vi "Insert2012.vi"(6 "Variant in":variant, 7 "Shift Pressed?":bool, 8 "error in (no error)":errorcluster, 10 "QD Combo Box Ref":refnum<vi>, 11 "QD Launch VI Ref":refnum<vi>) -> (0 "error out":errorcluster, 4 "Variant out":variant)   [LabVIEW 2012]
doc: "Inserts the object specified by name in the Quick Drop dialog box on the selected wire(s) on the diagram. If [Shift] is also pressed, and multiple wires were selected, a single instance of the object is inserted on those wires.\n\nDefault Shortcut - [I]"
uses:
  <vilib>/Utility/miscctls.llb/LVPositionTypeDef.ctl
  <vilib>/Utility/miscctls.llb/LVPointTypeDef.ctl
panel:
  in  "Style":i32(ring)=2125 items=[".NET Container"=2125, ".NET Refnum"=3441, "2D Picture"=3508, "3D Picture"=23776, "Absolute Value"=1054, "Access Rights"=1412, "ActiveX Container"=2072, "Add"=1050, "Add (with error terminals)"=3915, "Add Array Elements"=1903, "Agitator"=3831, "AllSpoll"=1960, "Always Copy"=2400, "And"=1061, "And Array Elements"=1911, "Append True/False String"=1511, "Application Refnum"=3412, "Array (block diagram constant)"=2070, "Array (classic)"=3300, "Array (modern)"=21608, "Array Interface Control"=23777, "Array Max & Min"=1907, "Array of Strings to Path"=1422, "Array Size"=1809, "Array Subset"=2044, "Array To Cluster"=1168, "Array To Spreadsheet String"=1540, "Atmospheric Tank (classic)"=3070, "Atmospheric Tank (modern)"=21751, "Automation Close"=8001, "Automation Open"=8000, "Automation Refnum"=3410, "Avogadro Constant (1/mol)"=23520, "Base 10 Logarithm Of e"=23512, "Bin #1"=3073, "Bin #2"=21755, "Bitpack to Array"=3135, "Bluetooth Close Connection"=9148, "Bluetooth Create Listener"=9151, "Bluetooth Discover"=9152, "Bluetooth Network Connection Refnum"=3468, "Bluetooth Open Connection"=9153, "Bluetooth Read"=9149, "Bluetooth Wait On Listener"=9147, "Bluetooth Write"=9150, "Boolean Array To Number"=1815, "Boolean To (0,1)"=1167, "Build Array"=2041, "Build Cluster Array"=2047, "Build Matrix"=8500, "Build Path"=1419, "Build Waveform"=2066, "Bundle"=2049, "Bundle By Name"=2057, "Byte Array To String"=1609, "Byte Stream File Refnum"=3408, "Call By Reference"=3901, "Call Chain"=1999, "Call Library Function Node"=2062, "Call Parent Method"=2354, "CAN Channel (block diagram constant)"=2124, "CAN Channel (classic)"=3340, "CAN Channel (modern)"=21817, "CAN Channel (system)"=21966, "CAN Interface (block diagram constant)"=2123, "CAN Interface (classic)"=3339, "CAN Interface (modern)"=21815, "CAN Interface (system)"=21964, "CAN Task (block diagram constant)"=3471, "CAN Task (classic)"=3470, "CAN Task (modern)"=21789, "CAN Task (system)"=21963, "Cancel Button (modern)"=21739, "Cancel Button (system)"=3131, "Cancel Notification"=9107, "Carriage Return Constant"=23500, "Case Structure"=2001, "Cast Unit Bases"=1079, "Check Valve"=3833, "Checkbox (classic)"=3117, "CheckBox (modern)"=21924, "Checkbox (system)"=3132, "Class Specifier Constant"=2094, "Clear Fixed-Point Overflow Status"=5562, "Close File"=8052, "Close File (deprecated)"=1405, "Close Reference"=8011, "Close Variable Connection"=23783, "Cluster (classic)"=3400, "Cluster (modern)"=21607, "Cluster Constant"=2071, "Cluster To Array"=1169, "Code Interface Node"=2050, "Coerce To Type"=2402, "Color Box"=3013, "Color Box Constant"=2120, "Color Box Thin Border"=2905, "Color Ramp"=3022, "Colored Rectangle (broken?)"=3625, "Combo Box (classic)"=3304, "Combo Box (modern)"=21604, "Combo Box (system)"=21917, "Combo Box Constant"=2088, "Complex Conjugate"=1048, "Complex To Polar"=1045, "Complex To Re/Im"=1044, "Compound Arithmetic"=2200, "Compressor"=3832, "Concatenate Strings"=2040, "Conditional Disable Structure"=2064, "Constructor Node"=3904, "Control & Simulation Loop"=2099, "Control Help Window"=1353, "Control Online Help"=1355, "Control Refnum"=3419, "Convert Unit"=2059, "Conveyer"=3827, "Copy"=8053, "Copy (deprecated)"=1416, "Cosecant"=1204, "Cosine"=1201, "Cotangent"=1205, "CPU Information"=24130, "Create Folder"=8055, "Create Network Stream Endpoint"=23793, "Create Network Stream Reader Endpoint"=23811, "Create Network Stream Writer Endpoint"=23810, "Create Stream"=23796, "Create Unique Network Stream Endpoint"=23795, "Create Unique Network Stream Reader Endpoint"=23807, "Create Unique Network Stream Writer Endpoint"=23806, "Create User Event"=2073, "Current Processor ID"=24131, "Current VI's Menubar"=9000, "Current VI's Path"=1426, "DAQmx Analog Trigger Source (block diagram constant)"=2119, "DAQmx Analog Trigger Source (classic)"=3336, "DAQmx Analog Trigger Source (modern)"=21774, "DAQmx Analog Trigger Source (system)"=21951, "DAQmx Device Name (block diagram constant)"=2093, "DAQmx Device Name (classic)"=3318, "DAQmx Device Name (modern)"=21773, "DAQmx Device Name (system)"=21950, "DAQmx Global Channel (block diagram constant)"=3430, "DAQmx Global Channel (classic)"=3443, "DAQmx Global Channel (modern)"=21770, "DAQmx Global Channel (system)"=21957, "DAQmx Physical Channel (block diagram constant)"=2118, "DAQmx Physical Channel (classic)"=3335, "DAQmx Physical Channel (modern)"=21777, "DAQmx Physical Channel (system)"=21954, "DAQmx Scale Name (block diagram constant)"=2116, "DAQmx Scale Name (classic)"=3317, "DAQmx Scale Name (modern)"=21775, "DAQmx Scale Name (system)"=21952, "DAQmx Switch (block diagram constant)"=2121, "DAQmx Switch (classic)"=3337, "DAQmx Switch (modern)"=21776, "DAQmx Switch (system)"=21953, "DAQmx Task Name (block diagram constant)"=3434, "DAQmx Task Name (classic)"=3442, "DAQmx Task Name (modern)"=21778, "DAQmx Task Name (system)"=21959, "DAQmx Terminal (block diagram constant)"=2117, "DAQmx Terminal (classic)"=3319, "DAQmx Terminal (modern)"=21781, "DAQmx Terminal (system)"=21955, "Data Cache Size"=24132, "Data Log File Refnum"=3402, "Data Value Reference"=3476, "Data Value Reference Constant"=24134, "DataSocket Close"=1085, "DataSocket Open"=1084, "DataSocket Read"=1086, "DataSocket Refnum"=3417, "DataSocket Write"=1087, "Date/Time To Seconds"=1308, "Decimal Digit?"=1119, "Decimal String To Number"=1184, "Decimate 1D Array"=2046, "DecomposeArray"=2412, "DecomposeLockDataValRef"=2406, "DecomposeVariant"=2404, "Decrement"=1058, "Default Directory"=1427, "Delete"=8056, "Delete (deprecated)"=1417, "Delete Data Value Reference"=2409, "Delete From Array"=3912, "Delete Menu Items"=9004, "Delete Variant Attribute"=8206, "Delete Waveform Attribute"=8209, "Deny Access"=8057, "Dequeue Element"=9113, "Destroy Stream Endpoint"=23794, "Destroy User Event"=2075, "DevClear"=1961, "DevClearList"=1962, "Device Control/Status"=1433, "Device Refnum"=3405, "Diagram Disable Structure"=2054, "Dial (classic)"=3050, "Dial (modern)"=21732, "Digital Data (classic)"=3210, "Digital Data (modern)"=21216, "Digital Waveform Graph (classic)"=3511, "Digital Waveform Graph (modern)"=21718, "Direct Variable Read"=23785, "Direct Variable Write"=23788, "Divide"=1053, "Divide (with error terminals)"=3918, "Dlg Horiz Scrollbar"=21905, "Dlg Numeric #1"=2100, "Dlg Numeric #2"=3006, "Dlg String"=2110, "Dlg Vert Scrollbar"=21906, "Down Arrow"=3824, "Down Bow Valve (flat)"=3707, "Down Bow Valve (outline)"=3807, "Down Bow Valve (shaded)"=21767, "Down Rect Valve (flat)"=3706, "Down Rect Valve (outline)"=3806, "Down Rect Valve (shaded)"=21766, "Down Tee (flat)"=3818, "Down Tee (shaded)"=3718, "Dynamic FPGA Interface Cast"=5690, "Elementary Charge (C)"=23517, "Empty Array?"=23063, "Empty Path Constant"=23523, "Empty String Constant"=23503, "Empty String/Path?"=1112, "Enable Menu Tracking"=9002, "EnableLocal"=1963, "EnableRemote"=1964, "End of Line Constant"=23525, "Enqueue Element"=9111, "Enqueue Element At Opposite End"=9129, "Enum (classic)"=3023, "Enum (modern)"=21605, "Enum (system)"=3062, "Enum Constant"=2090, "EOF"=1410, "Equal To 0?"=1113, "Equal?"=1102, "Error Ring Constant"=2039, "Event Callback Refnum"=3435, "Event Data Node"=2102, "Event Structure"=2052, "Exchanger"=3828, "Exclusive Or"=1063, "Exponential"=1211, "Exponential (Arg) -1"=1222, "Expression Node"=2201, "False Constant"=2006, "Feedback Node"=2353, "FieldPoint IO Point (block diagram constant)"=3440, "FieldPoint IO Point (classic)"=3439, "FieldPoint IO Point (modern)"=21784, "FIFO Refnum"=3474, "File Dialog"=8058, "File Dialog (deprecated)"=8081, "File Path Control (classic)"=3203, "File Path Control (modern)"=21730, "File Path Control (system)"=21922, "File Path Indicator (classic)"=3204, "File Path Indicator (modern)"=21731, "File/Directory Info"=8082, "File/Directory Info (deprecated)"=1413, "FindLstn"=1965, "FindRQS"=1966, "First Call?"=1083, "Fixed-Point Overflow?"=5565, "Fixed-Point to Integer Cast"=5566, "Flat Box"=3602, "Flat Circle"=3605, "Flat Down Triangle"=3623, "Flat Frame"=3608, "Flat Left Triangle"=3620, "Flat Right Triangle"=3621, "Flat Round Button"=3102, "Flat Rounded Box"=3611, "Flat Sequence Structure"=2069, "Flat Square Button"=3103, "Flat Up Triangle"=3622, "Flatten To JSON"=24201, "Flatten To String"=1164, "Flatten To XML"=8400, "Flattened String To Variant"=8202, "Floating Point Equal?"=23064, "Flush Event Queue"=2135, "Flush File"=8059, "Flush File (deprecated)"=1406, "Flush Queue"=9114, "Flush Stream"=23808, "For Loop"=2002, "Fork"=2194, "Format Date/Time String"=8100, "Format Into File"=2083, "Format Into String"=2081, "Format Value"=1512, "Formula Node"=2004, "FPGA Refnum to Session"=2322, "Fract/Exp String To Number"=1187, "Framed Color Box (classic)"=3008, "Framed Color Box (modern)"=21019, "Free Label"=2321, "Furnace"=3829, "Gauge (classic)"=3040, "Gauge (modern)"=21009, "Gauge for Simon"=32600, "Generate Front Panel Activity"=1329, "Generate Occurrence"=1700, "Generate User Event"=2074, "Generate User-Defined Trace Event"=2250, "Get Control Values by Index"=24204, "Get Datalog Position"=8061, "Get Date/Time In Seconds"=1303, "Get Date/Time String"=1600, "Get Drag Drop Data"=9154, "Get File Position"=8062, "Get File Size"=8063, "Get Fixed-Point Components"=11163, "Get Help Window Status"=1354, "Get Matrix Diagonal"=8501, "Get Matrix Elements"=8502, "Get Menu Item Info"=9005, "Get Menu Selection"=9001, "Get Menu Short Cut Info"=9007, "Get Notifier Status"=9103, "Get Number of Records"=8064, "Get Permissions"=8065, "Get Queue Status"=9110, "Get Submatrix"=8503, "Get Type and Creator"=8066, "Get Variant Attribute"=8205, "Get Volume Info"=8067, "Get Waveform Attribute"=8208, "Get Waveform Components"=2067, "Global Variable"=2060, "GPIB Clear"=1954, "GPIB Initialization"=1957, "GPIB Misc"=1956, "GPIB Read"=1951, "GPIB Serial Poll"=1955, "GPIB Status"=1959, "GPIB Trigger"=1953, "GPIB Wait"=1958, "GPIB Write"=1950, "Gravitational Constant (N m2/kg2)"=23519, "Greater Or Equal To 0?"=1114, "Greater Or Equal?"=1103, "Greater Than 0?"=1117, "Greater?"=1110, "Handle Peek"=1604, "Handle Poke"=1605, "Hex Digit?"=1123, "Hexadecimal String To Number"=1185, "Hopper #1"=21754, "Hopper #2"=3072, "Horiz Line"=3821, "Horiz Pipe (flat)"=3810, "Horiz Pipe (shaded)"=3710, "Horizontal Button Box"=3636, "Horizontal Fill Slide (classic)"=3012, "Horizontal Fill Slide (modern)"=21100, "Horizontal Gradient Oval"=32502, "Horizontal Gradient Rectangle"=32504, "Horizontal Gradient Rounded Rectangle"=32507, "Horizontal Graduated Bar"=21106, "Horizontal Pointer Slide (classic)"=3011, "Horizontal Pointer Slide (modern)"=21101, "Horizontal Pointer Slide (system)"=21902, "Horizontal Progress Bar (modern)"=21102, "Horizontal Progress Bar (system)"=21910, "Horizontal Scrollbar"=21110, "Horizontal Slide (classic)"=3010, "Horizontal Slide (system)"=21904, "Horizontal Slide Switch"=3114, "Horizontal Smooth Box"=3633, "Horizontal Splitter Bar"=21861, "Horizontal Splitter Bar (Classic)"=21863, "Horizontal Splitter Bar (System)"=21865, "Horizontal Switch"=3108, "Horizontal Tank"=3071, "Horizontal Toggle Switch (classic)"=3110, "Horizontal Toggle Switch (modern)"=21700, "Hyperbolic Cosecant"=23053, "Hyperbolic Cosine"=1215, "Hyperbolic Cotangent"=23055, "Hyperbolic Secant"=23054, "Hyperbolic Sine"=1214, "Hyperbolic Tangent"=1216, "IMAQ Session"=3415, "Implies"=1080, "In Place Element Structure"=2360, "In Range and Coerce"=1127, "Include Fixed-Point Overflow Status"=5564, "Increment"=1057, "Index & Bundle Cluster Array"=2056, "Index Array"=2042, "Index String Array"=1531, "Initialize Array"=2053, "Inline C Node"=2104, "Insert Into Array"=3911, "Insert Menu Items"=9003, "Integer to Fixed-Point Cast"=5567, "Intensity Chart (classic)"=3509, "Intensity Chart (modern)"=21719, "Intensity Graph (classic)"=3510, "Intensity Graph (modern)"=21720, "Interleave 1D Arrays"=2045, "Interpolate 1D Array"=1905, "Inverse Cosecant"=23050, "Inverse Cosine"=1207, "Inverse Cotangent"=23052, "Inverse Hyperbolic Cosecant"=23056, "Inverse Hyperbolic Cosine"=1218, "Inverse Hyperbolic Cotangent"=23058, "Inverse Hyperbolic Secant"=23057, "Inverse Hyperbolic Sine"=1217, "Inverse Hyperbolic Tangent"=1219, "Inverse Secant"=23051, "Inverse Sine"=1206, "Inverse Tangent"=1208, "Inverse Tangent (2 Input)"=1228, "Invoke Node"=3900, "IP To String"=1710, "IrDA Close Connection"=9144, "IrDA Create Listener"=9140, "IrDA Discover"=9141, "IrDA Network Connection Refnum"=3450, "IrDA Open Connection"=9142, "IrDA Read"=9145, "IrDA Wait On Listener"=9143, "IrDA Write"=9146, "IVI Delete Session"=8103, "IVI Logical Name (block diagram constant)"=3420, "IVI Logical Name (classic)"=3414, "IVI Logical Name (modern)"=21736, "IVI New Session"=8102, "Join"=2195, "Join Numbers"=1171, "Junction"=2197, "Knob (classic)"=3005, "Knob (modern)"=21000, "Label (modern)"=21960, "Label (system)"=21961, "Labeled Oblong Button"=3125, "Labeled Rectangular Button"=3124, "Labeled Round Button"=3122, "Labeled Square Button"=3123, "LabVIEW Object"=3457, "Leak Variant Value Reference"=2410, "LED Button"=3116, "Left Arrow"=3826, "Left Bow Valve (flat)"=3701, "Left Bow Valve (outline)"=3801, "Left Bow Valve (shaded)"=21761, "Left Down Elbow (flat)"=3811, "Left Down Elbow (shaded)"=3711, "Left Pump (flat)"=3813, "Left Pump (shaded)"=3713, "Left Rect Valve (flat)"=3700, "Left Rect Valve (outline)"=3800, "Left Rect Valve (shaded)"=21760, "Left Tee (flat)"=3809, "Left Tee (shaded)"=3709, "Left Up Elbow (flat)"=3808, "Left Up Elbow (shaded)"=3708, "Less Or Equal To 0?"=1115, "Less Or Equal?"=1104, "Less Than 0?"=1118, "Less?"=1111, "Lexical Class"=1126, "Line (chiseled, system)"=3632, "Line (chiseled, thick)"=3630, "Line (chiseled, thin)"=3627, "Line (thick)"=3629, "Line (thin)"=3626, "Line Feed Constant"=23501, "Line with Arrow (thick)"=3631, "Line with Arrow (thin)"=3628, "List Directory"=1418, "List Folder"=8083, "Listbox (classic)"=21806, "Listbox (modern)"=21792, "Listbox (system)"=21805, "Listbox Symbol Ring Constant"=2038, "Local Variable"=2061, "Lock Range"=1411, "Logarithm Base 10"=1210, "Logarithm Base 2"=1225, "Logarithm Base X"=1224, "Logical Shift"=1081, "Lossy Enqueue Element"=9130, "Lowered Box (thick)"=3635, "Lowered Rounded Box"=3638, "Machine Epsilon"=23528, "MakeAddr"=1967, "Mantissa & Exponent"=1150, "Match First String"=1532, "Match Pattern"=1535, "Match True/False String"=1533, "MathScript Call By Reference"=3906, "MathScript Node"=2357, "MATLAB script"=9020, "Matrix Size"=8507, "Max & Min"=1108, "Menu Refnum"=3413, "Menu Ring (classic)"=3018, "Menu Ring (modern)"=21600, "Menu-Popup Ring"=3017, "Merge Errors"=2147, "Merge Signals"=2350, "Meter (classic)"=3030, "Meter (modern)"=21008, "Mixed Checkbox (system)"=21333, "Mixed Signal Graph"=21721, "Molar Gas Constant (J/(mol K))"=23522, "Motion Resource (block diagram constant)"=3449, "Motion Resource (classic)"=3448, "Motion Resource (modern)"=21787, "Motor (flat)"=3820, "Motor (shaded)"=3720, "Move"=8068, "Move (deprecated)"=1415, "Multi-Segment Pipe"=23780, "Multicolumn Listbox (classic)"=21799, "Multicolumn Listbox (modern)"=21791, "Multicolumn Listbox (system)"=21798, "Multiply"=1052, "Multiply (with error terminals)"=3917, "Multiply Array Elements"=1904, "Multirate Structure"=2199, "Natural Logarithm"=1209, "Natural Logarithm (Arg +1)"=1221, "Natural Logarithm Base"=23510, "Natural Logarithm Of 10"=23513, "Natural Logarithm Of 2"=23514, "Natural Logarithm Of Pi"=23508, "Negate"=1069, "Negative Infinity"=23509, "New Data Value Reference"=2408, "New Directory"=1402, "New File"=1404, "New VI"=8014, "New VI Object"=8015, "Not"=1064, "Not A Number/Path/Refnum?"=1128, "Not A Path Constant"=23524, "Not a Refnum Constant"=23526, "Not a Shared Variable"=23527, "Not And"=1071, "Not Equal To 0?"=1116, "Not Equal?"=1105, "Not Exclusive Or"=1073, "Not Or"=1072, "Notifier Refnum"=3423, "Number of Cache Levels"=24133, "Number To Boolean Array"=1814, "Number To Decimal String"=1180, "Number To Engineering String"=1183, "Number To Exponential String"=1505, "Number To Fractional String"=1506, "Number To Hexadecimal String"=1181, "Number To Octal String"=1182, "Numeric Constant"=2005, "Numeric Control (classic)"=3000, "Numeric Control (modern)"=21003, "Numeric Control (system)"=21919, "Numeric Indicator (classic)"=3001, "Numeric Indicator (modern)"=21004, "Obtain Notifier"=9101, "Obtain Queue"=9108, "Occurrence Refnum"=3406, "Octal Digit?"=1129, "Octal String To Number"=1186, "OK Button (modern)"=21738, "OK Button (system)"=3130, "Old VISA Open"=1921, "OLE Variant"=3150, "One Button Dialog"=1340, "Open and Verify Variable Connection"=23790, "Open Application Reference"=8012, "Open Device"=1430, "Open Dynamic Bitfile Reference"=5691, "Open File"=1403, "Open Tank (flat classic)"=21752, "Open Tank (shaded classic)"=3074, "Open Variable Connection"=23779, "Open Variable Connection in Background"=23791, "Open VI Object Reference"=8013, "Open VI Reference"=8010, "Open/Create/Replace Datalog"=8054, "Open/Create/Replace File"=8050, "Or"=1062, "Or Array Elements"=1910, "Oval with Shadow"=32509, "Package Matrix"=23001, "PassControl"=1968, "Path Constant"=2009, "Path to Array of Strings"=1423, "Path To String"=1077, "Path Type"=1421, "Pi"=23504, "Pi Divided By 2"=23506, "Pi Multiplied By 2"=23505, "Pick Line"=1510, "Pict Ring (classic)"=3015, "Pict Ring (modern)"=21602, "Pict Ring (system)"=21925, "PixMap"=3505, "PixMap (warning: dangerous)"=3507, "Planck's Constant (J/Hz)"=23516, "Platform Flat Square Button"=3134, "Plug-In Control"=21820, "Polar To Complex"=1047, "Polar To Re/Im"=23061, "Positive Infinity"=23515, "Power Of 10"=1212, "Power Of 2"=1223, "Power Of X"=1213, "PPoll"=1969, "PPollConfig"=1970, "PPollUnconfig"=1971, "Preallocated Read from Binary File"=24135, "Preserve Run-Time Class"=8018, "Pressure Tank (flat)"=3075, "Pressure Tank (shaded)"=21753, "Preview Queue Element"=9112, "Printable?"=1124, "Property Node"=1920, "Pulldown Menu Ring"=3061, "Push Button"=21001, "Queue Refnum"=3424, "Quit LabVIEW"=1352, "Quotient & Remainder"=1056, "Radio Button (system)"=3133, "Radio Buttons (classic)"=22003, "Radio Buttons (modern)"=22001, "Radio Buttons (system)"=22002, "Raised Box (classic)"=3600, "Raised Box (modern)"=3637, "Raised Circle"=3603, "Raised Down Triangle"=3615, "Raised Frame"=3606, "Raised Left Triangle"=3612, "Raised Right Triangle"=3613, "Raised Rounded Box"=3609, "Raised Up Triangle"=3614, "Random Number (0-1)"=1070, "RcvRespMsg"=1972, "Re/Im To Complex"=1046, "Re/Im To Polar"=23060, "Read Datalog"=8069, "Read Device"=1432, "Read File"=1407, "Read from Binary File"=8051, "Read from Text File"=8070, "Read Multiple Elements from Stream"=23803, "Read Single Element from Stream"=23797, "Read Variable"=23781, "Read Variable with Timeout"=23786, "ReadStatus"=1973, "Receive"=1974, "ReceiveSetup"=1975, "Recessed Box"=3601, "Recessed Circle"=3604, "Recessed Down Triangle"=3619, "Recessed Frame (modern)"=3607, "Recessed Frame (system)"=3624, "Recessed Left Triangle"=3616, "Recessed Menu Ring"=3019, "Recessed Right Triangle"=3617, "Recessed Rounded Box"=3610, "Recessed Up Triangle"=3618, "Reciprocal"=1059, "Reciprocal Of e"=23511, "Reciprocal Of Pi"=23507, "RecomposeArray"=2403, "RecomposeUnlockDataValRef (warning: dangerous)"=2407, "RecomposeVariant (warning: dangerous)"=2405, "Rectangular Stop Button"=3128, "Refnum to Path"=1424, "Refnum to Session"=2306, "Region"=2196, "Register Event Callback"=2078, "Register For Events"=2065, "Register Session"=2319, "Release Notifier"=9102, "Release Queue"=9109, "Remove Fixed-Point Overflow Status"=5563, "Replace Array Subset"=3910, "Replace Substring"=3913, "Request Deallocation"=1610, "ResetSys"=1976, "Reshape Array"=2055, "Resize Matrix"=8508, "Resource Index"=1088, "Reverse 1D Array"=1900, "Reverse String"=1537, "Right Arrow"=3825, "Right Bow Valve (flat)"=3705, "Right Bow Valve (outline)"=3805, "Right Bow Valve (shaded)"=21765, "Right Down Elbow (flat)"=3817, "Right Down Elbow (shaded)"=3717, "Right Pump (flat)"=3819, "Right Pump (shaded)"=3719, "Right Rect Valve (flat)"=3704, "Right Rect Valve (outline)"=3804, "Right Rect Valve (shaded)"=21764, "Right Tee (flat)"=3815, "Right Tee (shaded)"=3715, "Right Up Elbow (flat)"=3814, "Right Up Elbow (shaded)"=3714, "Rocker"=21002, "Rotary Feeder"=3830, "Rotate"=1082, "Rotate 1D Array"=1906, "Rotate Left With Carry"=1606, "Rotate Right With Carry"=1607, "Rotate String"=1536, "Round Button"=3100, "Round LED (classic)"=3120, "Round LED (modern)"=21012, "Round Light"=3104, "Round Push Button"=3118, "Round Push Button (profile)"=3112, "Round Radio Button"=3106, "Round Stop Button"=3127, "Round To Nearest"=1055, "Round Toward +Infinity"=1076, "Round Toward -Infinity"=1075, "Rounded Rectangle with Shadow"=32508, "RT FIFO Create"=24000, "RT FIFO Delete"=24003, "RT FIFO Read"=24001, "RT FIFO Write"=24002, "Rydberg Constant (1/m)"=23521, "Scale By Power Of 2"=1074, "Scan From File"=2082, "Scan From String"=2080, "Scan String For Tokens"=8101, "Scan Value"=1534, "Scanned Variable Read"=23784, "Scanned Variable Write"=23787, "Search 1D Array"=1901, "Search and Replace String"=3914, "Search Variable Container"=23802, "Search/Split String"=1538, "Secant"=1203, "Seconds To Date/Time"=1309, "Seek"=1409, "Select"=1516, "Send"=1977, "Send Notification"=9104, "SendCmds"=1978, "SendDataBytes"=1979, "SendIFC"=1980, "SendList"=1981, "SendLLO"=1982, "SendSetup"=1983, "Session to Refnum"=2307, "Set Control Values by Index"=24203, "Set Datalog Position"=8072, "Set File Position"=8073, "Set File Size"=8074, "Set Matrix Diagonal"=8504, "Set Matrix Elements"=8505, "Set Menu Item Info"=9006, "Set Number of Records"=8075, "Set Occurrence"=1702, "Set Permissions"=8076, "Set Submatrix"=8506, "Set Type and Creator"=8077, "Set Variant Attribute"=8204, "Set Waveform Attribute"=8207, "SetRWLS"=1984, "SetTimeOut"=1985, "Shared Variable"=23778, "Shared Variable Constant"=3473, "Shared Variable Control (classic)"=3472, "Shared Variable Control (modern)"=21814, "Shared Variable to String"=1831, "Sign"=1049, "Simple Horizontal Slide"=3003, "Simple Numeric"=2900, "Simple String"=2115, "Simple Vertical Slide"=3002, "Sinc"=1227, "Sine"=1200, "Sine & Cosine"=1220, "Size Handle"=1603, "Slide Switch"=21011, "Smoothed Oval"=32500, "Smoothed Rounded Rectangle"=32505, "Sort 1D Array"=1120, "Sort Array of String"=23065, "Speed Of Light In Vacuum (m/sec)"=23518, "Spin Control (system)"=21900, "Split 1D Array"=1908, "Split Button"=21020, "Split Number"=1170, "Split Signals"=2351, "Spreadsheet String To Array"=1539, "Square"=23059, "Square Button"=3101, "Square LED (classic)"=3121, "Square LED (modern)"=21013, "Square Light"=3105, "Square Push Button"=3119, "Square Push Button (profile)"=3113, "Square Radio Button"=3107, "Square Root"=1060, "Stacked Sequence Structure"=2000, "State"=2198, "State Diagram"=2051, "Static VI Reference"=2084, "Stop"=1350, "Stop Button"=21230, "String Constant"=2007, "String Control (classic)"=3200, "String Control (modern)"=21701, "String Control (system)"=21920, "String Indicator (classic)"=3201, "String Indicator (modern)"=21702, "String Length"=1502, "String Subset"=1503, "String To Byte Array"=1608, "String To IP"=1711, "String To Path"=1078, "String to Shared Variable"=1830, "Strip Path"=1420, "SubPanel"=21810, "SubPanel (Classic)"=21811, "SubPanel (System)"=21823, "Subtract"=1051, "Subtract (with error terminals)"=3916, "Swap Bytes"=1162, "Swap Values"=2401, "Swap Vector Element"=1912, "Swap Words"=1163, "Tab Constant"=23502, "Tab Control (classic)"=3330, "Tab Control (modern)"=3332, "Tab Control (system)"=3331, "Table (classic)"=21796, "Table (modern)"=21790, "Table (system)"=21797, "Tag Attribute Ring"=2063, "Tangent"=1202, "Tank (classic)"=3020, "Tank (modern)"=21006, "TCP Close Connection"=1713, "TCP Create Listener"=1717, "TCP Flattened Read"=1718, "TCP Flattened Write"=1719, "TCP Flex Read"=1720, "TCP Flex Write"=1721, "TCP Network Connection Refnum"=3407, "TCP Open Connection"=1715, "TCP Read"=1716, "TCP Wait On Listener"=1712, "TCP Write"=1714, "TDMS Advanced Asynchronous Read (Data Ref)"=2151, "TDMS Advanced Asynchronous Write (Data Ref)"=2150, "TDMS Close"=24113, "TDMS Configure Asynchronous Reads (Data Ref)"=2153, "TDMS Configure Asynchronous Writes (Data Ref)"=2152, "TDMS Defragment"=24119, "TDMS File"=3477, "TDMS Flush"=24117, "TDMS Get Asynchronous Read Status (Data Ref)"=2155, "TDMS Get Asynchronous Write Status (Data Ref)"=2154, "TDMS Get Properties"=24115, "TDMS In Memory Close"=2157, "TDMS In Memory Open"=2156, "TDMS In Memory Read Bytes"=2158, "TDMS List Contents"=24116, "TDMS Open"=24112, "TDMS Read"=24111, "TDMS Refnum To File ID"=24120, "TDMS Set Properties"=24114, "TDMS Write"=24110, "TDMS Write IP"=24118, "Temporary Directory"=1435, "TestSRQ"=1986, "TestSys"=1987, "Text & Pict Ring (classic)"=3016, "Text & Pict Ring (modern)"=21603, "Text Button"=21015, "Text Ring (block diagram constant)"=2008, "Text Ring (classic)"=3014, "Text Ring (modern)"=21601, "Text Ring (system)"=3060, "Text to UTF-8"=23066, "Thermometer (classic)"=3021, "Thermometer (modern)"=21007, "Threshold 1D Array"=1909, "Tick Count (ms)"=1300, "Time Stamp (block diagram constant)"=2068, "Time Stamp Control (classic)"=5555, "Time Stamp Control (modern)"=21913, "Time Stamp Control (system)"=21967, "Time Stamp Indicator (classic)"=5556, "Time Stamp Indicator (modern)"=21914, "Timed Loop"=5570, "Timed Sequence"=5573, "To Byte Integer"=1140, "To Double Precision Complex"=1152, "To Double Precision Float"=1147, "To Extended Precision Complex"=1154, "To Extended Precision Float"=1149, "To Fixed-Point"=5561, "To Long Integer"=1142, "To Lower Case"=1189, "To More Generic Class"=8017, "To More Specific Class"=8016, "To OLE Variant"=8002, "To Probe String"=2413, "To Quad Integer"=1155, "To Single Precision Complex"=1151, "To Single Precision Float"=1146, "To Time Stamp"=5560, "To Unsigned Byte Integer"=1143, "To Unsigned Long Integer"=1145, "To Unsigned Quad Integer"=1156, "To Unsigned Word Integer"=1144, "To Upper Case"=1188, "To Variant"=8201, "To Word Integer"=1141, "Traditional DAQ Channel (block diagram constant)"=2085, "Traditional DAQ Channel (classic)"=3320, "Traditional DAQ Channel (modern)"=21733, "Transpose 1D Array"=23068, "Transpose 2D Array"=1902, "Transpose Matrix"=8509, "Tree (classic)"=21819, "Tree (modern)"=21793, "Tree (system)"=21794, "Trigger"=1988, "TriggerList"=1989, "Two Button Dialog"=1341, "Type and Creator"=1434, "Type Cast"=1166, "UDP Close"=1726, "UDP Multicast Open"=1727, "UDP Network Connection Refnum"=3418, "UDP Open"=1723, "UDP Read"=1724, "UDP Write"=1725, "Unbitpack from Array"=3136, "Unbundle"=2048, "Unbundle By Name"=2058, "Unflatten From JSON"=24202, "Unflatten From String"=1165, "Unflatten From XML"=8401, "Unleak Variant Value Reference"=2411, "Unpackage Matrix"=23000, "Unregister For Events"=2076, "Unregister Session"=2320, "Up Arrow"=3823, "Up Bow Valve (flat)"=3703, "Up Bow Valve (outline)"=3803, "Up Bow Valve (shaded)"=21763, "Up Rect Valve (flat)"=3702, "Up Rect Valve (outline)"=21762, "Up Rect Valve (shaded)"=3802, "Up Tee (flat)"=3812, "Up Tee (shaded)"=3712, "User Defined Refnum"=3428, "User Defined Refnum Tag (block diagram constant)"=3426, "User Defined Refnum Tag (classic)"=3429, "User Defined Refnum Tag (modern)"=21745, "User Defined Refnum Tag Flatten (classic)"=3454, "User Defined Refnum Tag Flatten (modern)"=21747, "User Defined Tag (block diagram constant)"=2114, "User Defined Tag (classic)"=3329, "User Defined Tag (modern)"=21749, "User Item"=3506, "UTF-8 to Text"=23067, "Variable Class Specifier Constant"=2106, "Variable Name Constant"=3478, "Variant"=3310, "Variant To Data"=8003, "Variant To Flattened String"=8203, "Vert Line"=3822, "Vert Pipe (flat)"=3816, "Vert Pipe (shaded)"=3716, "Vert Rocker"=21740, "Vertical Fill Slide (classic)"=3009, "Vertical Fill Slide (modern)"=21014, "Vertical Gradient Oval"=32501, "Vertical Gradient Rectangle"=32503, "Vertical Gradient Rounded Rectangle"=32506, "Vertical Graduated Bar"=21107, "Vertical Pointer Slide (classic)"=3007, "Vertical Pointer Slide (modern)"=21017, "Vertical Pointer Slide (system)"=21901, "Vertical Progress Bar (modern)"=21104, "Vertical Progress Bar (system)"=21909, "Vertical Scrollbar"=21111, "Vertical Slide"=3004, "Vertical Slide (system)"=21903, "Vertical Slide Switch (classic)"=3115, "Vertical Slide Switch (modern)"=21741, "Vertical Smooth Box"=3634, "Vertical Splitter Bar"=21860, "Vertical Splitter Bar (Classic)"=21862, "Vertical Splitter Bar (System)"=21864, "Vertical Switch"=3109, "Vertical Toggle Switch (classic)"=3111, "Vertical Toggle Switch (modern)"=21005, "VI Library"=1425, "VI Refnum"=3422, "VI Server Reference"=2091, "VISA Assert Interrupt Signal"=2309, "VISA Assert Trigger"=1929, "VISA Assert Utility Signal"=2310, "VISA Clear"=1927, "VISA Close"=1922, "VISA Disable Event"=1940, "VISA Discard Events"=1941, "VISA Enable Event"=1942, "VISA Find Resource"=1923, "VISA Flush I/O Buffer"=2302, "VISA GPIB Command"=2315, "VISA GPIB Control ATN"=2316, "VISA GPIB Control REN"=2304, "VISA GPIB Pass Control"=2317, "VISA GPIB Send IFC"=2318, "VISA In 16"=1930, "VISA In 32"=1944, "VISA In 64"=2140, "VISA In 8"=1936, "VISA Lock"=1993, "VISA Map Address"=1932, "VISA Map Trigger"=2311, "VISA Memory Allocation"=1997, "VISA Memory Allocation Ex"=2146, "VISA Memory Free"=1998, "VISA Move"=2303, "VISA Move In 16"=1948, "VISA Move In 32"=1991, "VISA Move In 64"=2144, "VISA Move In 8"=1946, "VISA Move Out 16"=1949, "VISA Move Out 32"=1992, "VISA Move Out 64"=2145, "VISA Move Out 8"=1947, "VISA Open"=2308, "VISA Out 16"=1931, "VISA Out 32"=1945, "VISA Out 64"=2141, "VISA Out 8"=1937, "VISA Peek 16"=1934, "VISA Peek 32"=1995, "VISA Peek 64"=2142, "VISA Peek 8"=1938, "VISA Poke 16"=1935, "VISA Poke 32"=1996, "VISA Poke 64"=2143, "VISA Poke 8"=1939, "VISA Read"=1925, "VISA Read STB"=1928, "VISA Read To File"=2313, "VISA Refnum to Session"=2300, "VISA Resource Name"=3421, "VISA resource name (classic)"=3409, "VISA resource name (modern)"=21737, "VISA Set I/O Buffer Size"=2301, "VISA Status Description"=1924, "VISA Unlock"=1994, "VISA Unmap Address"=1933, "VISA Unmap Trigger"=2312, "VISA USB Control In"=2086, "VISA USB Control Out"=2087, "VISA VXI Cmd or Query"=2305, "VISA Wait on Event"=1943, "VISA Write"=1926, "VISA Write From File"=2314, "Volume Info"=1414, "Wait (ms)"=1302, "Wait For Activity"=1722, "Wait For Front Panel Activity"=1328, "Wait for GPIB RQS"=1952, "Wait on Notification"=9105, "Wait on Notification from Multiple"=9106, "Wait on Notification from Multiple with Notifier History"=9132, "Wait on Notification with Notifier History"=9131, "Wait on Occurrence"=1701, "Wait Until Next ms Multiple"=1327, "WaitSRQ"=1990, "Waveform Chart"=21010, "Waveform Chart (classic)"=3501, "Waveform Chart (modern)"=21717, "Waveform Graph (classic)"=3504, "Waveform Graph (modern)"=21703, "While Loop #1"=2003, "While Loop #2"=2352, "White Space?"=1125, "Write Datalog"=8079, "Write Device"=1431, "Write File"=1408, "Write Multiple Elements to Stream"=23804, "Write Single Element to Stream"=23798, "Write to Binary File"=8078, "Write to Text File"=8080, "Write Variable"=23782, "Write Variable with Timeout"=23789, "XY Graph (classic)"=3500, "XY Graph (modern)"=21716, "Y-th Root of X"=23062]
  in  "Undo Name":string="Insert"
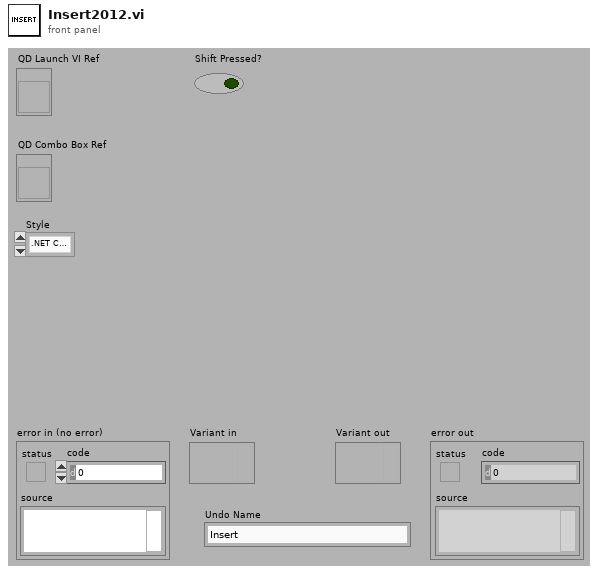
[diagram p1: front panel]
types:
  T1 = cluster{"Not Error Wire?":bool, "Source Term Top":i32, "Source Term Left":i32, "Wire Ref":refnum<vi>, "Source Term":refnum<vi>, "Sink Terms":refnum<vi>[], "Tried this one yet?":bool, "Sink Term Owner Owners":refnum<vi>[]}
  T2 = typedef "LVPositionTypeDef.ctl" = cluster{"Left":i32, "Top":i32}
  T3 = typedef "LVPointTypeDef.ctl" = cluster{"Horizontal":i16, "Vertical":i16}
  T4 = cluster{"Position":cluster{"h":i16, "v":i16}, "Flags":i32, "Type":enum32{"LooseEnd", "Endpoint", "Bend", "Junction"}, "Up Joint Index":i16, "Down Joint Index":i16, "Left Joint Index":i16, "Right Joint Index":i16}[]
  T5 = cluster{"Joints[]":cluster{"Position":cluster{"h":i16, "v":i16}, "Flags":i32, "Type":enum32{"LooseEnd", "Endpoint", "Bend", "Junction"}, "Up Joint Index":i16, "Down Joint Index":i16, "Left Joint Index":i16, "Right Joint Index":i16}[]}
  T6 = typedef "LVStringsAndValuesArrayTypeDef_I32.ctl" = cluster{"String":string, "Value":i32}[]
  T7 = cluster{"Not Error Wire?":bool, "Source Term Top":i32, "Source Term Left":i32, "Wire Ref":refnum<vi>, "Source Term":refnum<vi>, "Sink Terms":refnum<vi>[], "Tried this one yet?":bool, "Sink Term Owner Owners":refnum<vi>[]}[]
  T8 = cluster{"Position":cluster{"h":i16, "v":i16}, "Flags":i32, "Type":enum32{"LooseEnd", "Endpoint", "Bend", "Junction"}, "Up Joint Index":i16, "Down Joint Index":i16, "Left Joint Index":i16, "Right Joint Index":i16}
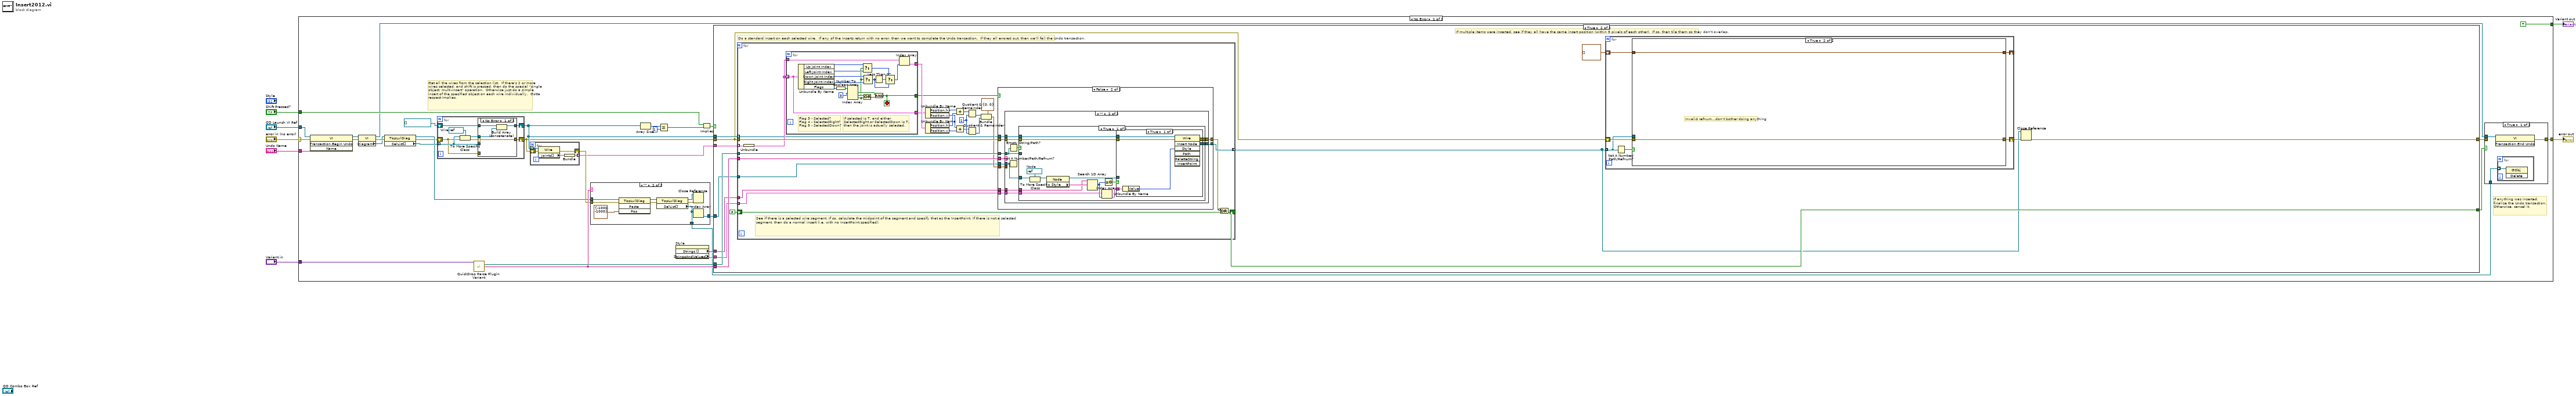
[diagram p0: block diagram]
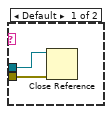
[diagram p2: hidden frame]
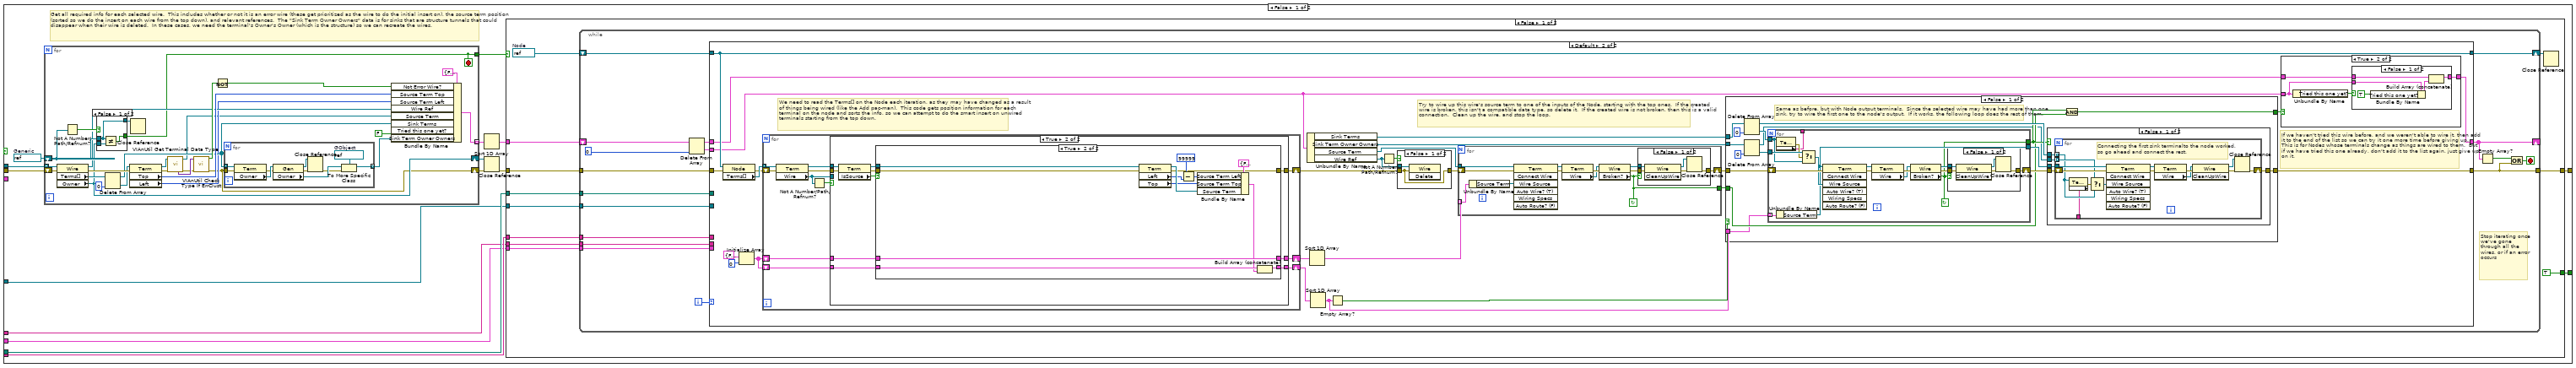
[diagram p3: hidden frame]
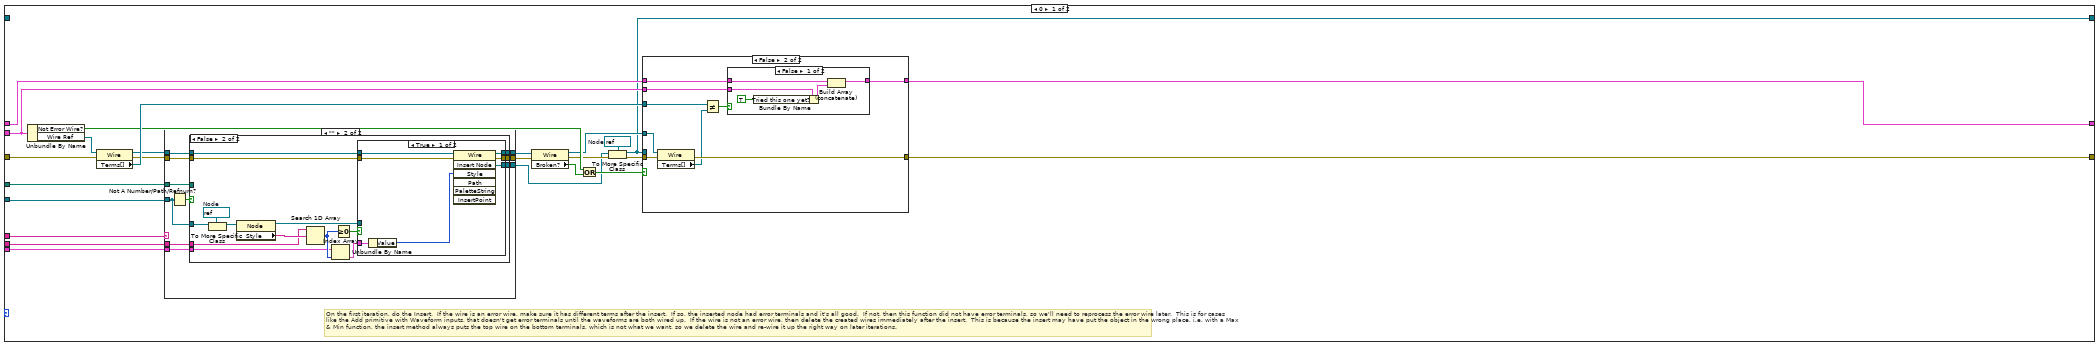
[diagram p4: hidden frame]
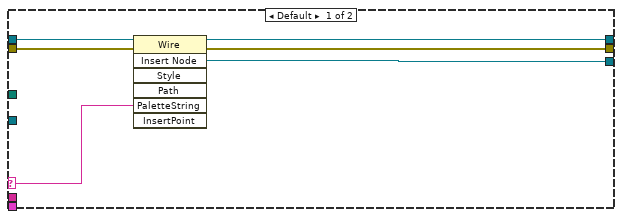
[diagram p5: hidden frame]
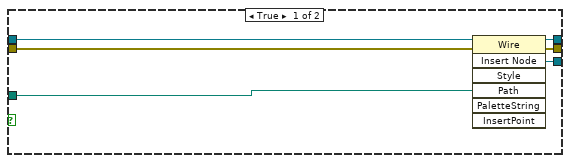
[diagram p6: hidden frame]
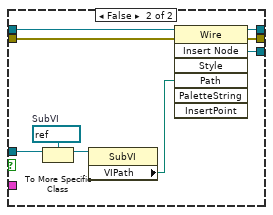
[diagram p7: hidden frame]
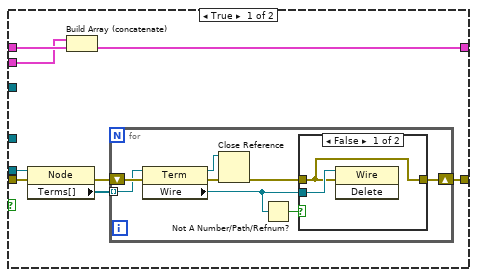
[diagram p8: hidden frame]
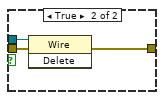
[diagram p13: hidden frame]
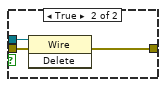
[diagram p17: hidden frame]
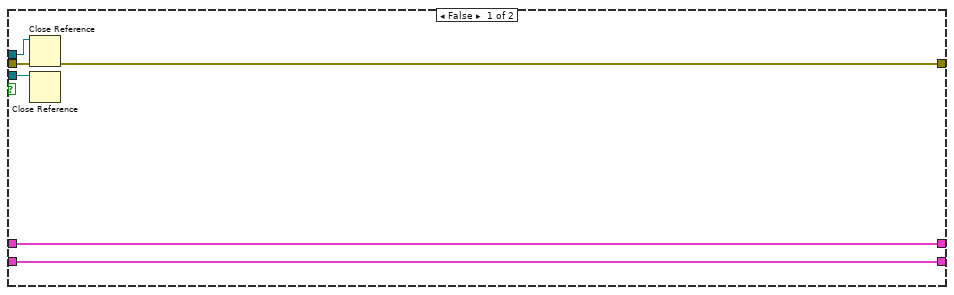
[diagram p18: hidden frame]
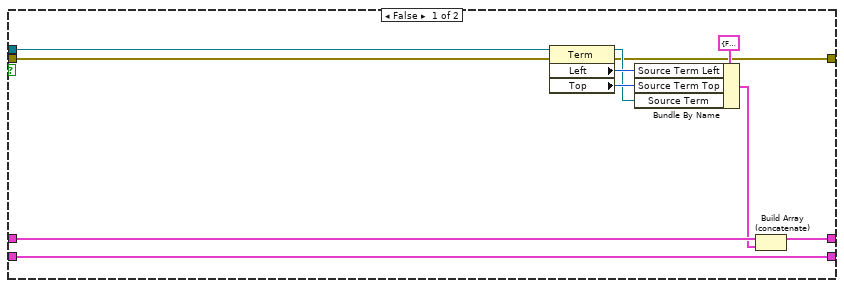
[diagram p19: hidden frame]
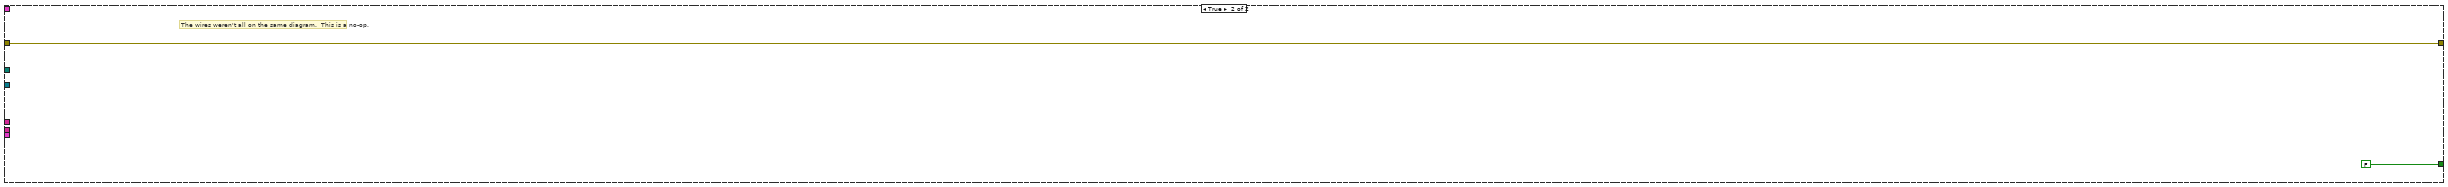
[diagram p20: hidden frame]
diagram:
  n1 = case shown="No Error" "error in (no error)" {
    selector: "error in (no error)" -> [w38 w683]
    tunnel: [w33 w683] -> w6
    tunnel: "QD Launch VI Ref" -> [w37 _]
    tunnel: "Shift Pressed?" -> [w25 _]
    tunnel: "Variant in" -> [w39 _]
    tunnel: "Undo Name" -> [w36 _]
    tunnel: [TRUE _] -> w1
    frame No Error {
      # "If anything was inserted, finalize the Undo transaction.  Otherwise, cancel it."
      # "Get all the wires from the selection list.  If there's 2 or more wires selected, and shift is pressed, then do the special \"single object, multi-insert\" operation.  Otherwise just do a simple insert of the specified object on each wire individually.  Gotta respect Implies."
      n2 = invoke class="VI" method="Transaction.Begin Undo"(reference=w37, error in=w38, "Name"=w36) -> (reference out=w20:refnum<vi>, error out=w34:errorcluster)  [unwired: 1 in, 2 out]
      n3 = property class="VI"(reference=w20, error in=w34) -> (reference out=w19:refnum<vi>, error out=w32:errorcluster, "Diagram"=w31:refnum<vi>)
      n4 = property class="TopLvlDiag"(reference=w31, error in=w32) -> (reference out=w17:refnum<vi>, error out=w16:errorcluster, "SelList[]"=w30:refnum<vi>[])
      n5 = for {
        tunnel: w30 -> [w666] mode=indexing
        shift-right: [w665] -> w11
        shift-left: refnum<vi>[] [] -> [w667]
        shift-right: [w663] -> w10
        shift-left: w16 -> [w662]
        w669 = refnum<vi> refnum  # Wire
        n6 = To More Specific Class(target class=w669, reference=w666, error in=w662) -> (specific class reference=w664:refnum<vi>, error out=w668:errorcluster)
        n7 = case shown="No Error" w668 {
          selector: w668 -> [w670 _]
          tunnel: w667 -> [w673 w676]
          tunnel: w666 -> [_ w675]
          tunnel: [w672 w676] -> w665
          tunnel: w664 -> [w671 _]
          tunnel: [w670 w674] -> w663
          tunnel: w662 -> [_ w674]
          frame No Error {
            n8 = Build Array (concatenate)(w673, w671) -> (w672:refnum<vi>[])
          }
          frame Error {
            n9 = Close Reference(reference=w675) -> ()  [unwired: 1 in, 1 out]
          }
        }
      }
      n10 = call <vilib>:"QuickDrop Parse Plugin Variant.vi"("QDKS Variant in"=w39) -> ("Project VI Path"=w24:path, "Palette Object Name"=w18:string)  [unwired: 12 in, 1 out]
      n11 = for {
        tunnel: w11 -> [w44] mode=indexing
        tunnel: [w42] -> w8 mode=indexing
        shift-right: [w40] -> w9
        shift-left: w10 -> [w41]
        n12 = property class="Wire"(reference=w44, error in=w41) -> (error out=w40:errorcluster, "Joints[]"=w43:T4)  [unwired: 1 out]
        n13 = Bundle("Joints[]"=w43) -> (w42:T5)  [unwired: 1 in]
      }
      n14 = case shown="\"\"" w18 {
        tunnel: [_ w49] -> w12
        tunnel: w17 -> [w46 w52]
        tunnel: w9 -> [w45 w50]
        tunnel: [_ w47] -> w13
        frame Default {
          n15 = Close Reference(reference=w46, error in (no error)=w45) -> ()  [unwired: 1 out]
        }
        frame "" {
          n16 = invoke class="TopLvlDiag" method="Paste"(reference=w52, error in=w50, "Pos"=cluster{"Left":i32, "Top":i32} {"Left"=-1000, "Top"=-1000}) -> (reference out=w51:refnum<vi>, error out=w53:errorcluster)  [unwired: 1 in, 2 out]
          n17 = property class="TopLvlDiag"(reference=w51, error in=w53) -> (reference out=w54:refnum<vi>, error out=w55:errorcluster, "SelList[]"=w47:refnum<vi>[])
          n18 = Close Reference(reference=w54, error in (no error)=w55) -> ()  [unwired: 1 out]
          n19 = Index Array(array=w47) -> (element=w49:refnum<vi>)  [unwired: 1 in]
        }
      }
      n20 = Array Size(array=w11) -> (size(s)=w28:i32)
      n21 = Less Or Equal?(x=w28, y=1) -> (x <= y?=w26:bool)
      n22 = property on="Style" class="Ring (strict)"() -> ("Strings []"=w15:string[], "StringsAndValues[]"=w14:T6)  [unwired: 2 in, 2 out]
      n23 = Implies(1:w26, 2:w25) -> (0:w23:bool)
      n24 = case shown="True" w23 {
        tunnel: w18 -> [w61 w441]
        tunnel: w24 -> [w62 w440]
        tunnel: w11 -> [w67 w439]
        tunnel: w10 -> [w66 w432]
        tunnel: [w60 w435] -> w22
        tunnel: [w59 w437] -> w21
        tunnel: w12 -> [w58 w431]
        tunnel: w15 -> [w57 w430]
        tunnel: w14 -> [w56 w429]
        tunnel: w8 -> [_ w428]
        frame False {
          w70 = refnum<vi> refnum  # Generic
          # "Get all required info for each selected wire.  This includes whether or not it is an error wire (these get prioritized as the wire to do the initial insert on), the source term position (sorted so we do the insert on each wire from the top down), and relevant references.  The \"Sink Term Owner Owners\" data is for sinks that are structure tunnels that could disappear when their wire is deleted.  In these cases, we need the terminal's Owner's Owner (which is the structure) so we can recreate the wires."
          n25 = for {
            shift-right: [w392] -> w64
            shift-left: w66 -> [w413]
            shift-right: [w396] -> w71
            shift-left: w70 -> [w412]
            tunnel: [w397] -> w69
            tunnel: w67 -> [w400] mode=indexing
            tunnel: [w399] -> w65 mode=indexing
            stop <- w397 stop-if-true
            n26 = property class="Wire"(reference=w400, error in=w413) -> (reference out=w403:refnum<vi>, error out=w409:errorcluster, "Terms[]"=w411:refnum<vi>[], "Owner"=w396:refnum<vi>)
            n27 = Not A Number/Path/Refnum?(number/path/refnum=w412) -> (NaN/Path/Refnum?=w408:bool)
            n28 = case shown="False" w408 {
              tunnel: [w425 FALSE] -> w397
              tunnel: w396 -> [w426 _]
              tunnel: w412 -> [w424 _]
              tunnel: [w424 _] -> w393
              frame False {
                n29 = Not Equal?(x=w424, y=w426) -> (x != y?=w425:bool)
              }
              frame True {
              }
            }
            n30 = Delete From Array(array=w411, index=0) -> (deleted portion=w398:refnum<vi>, array with subset deleted=w395:refnum<vi>[])  [unwired: 1 in]
            n31 = property class="Term"(reference=w398, error in=w409) -> (reference out=w390:refnum<vi>, error out=w391:errorcluster, "Top"=w405:i32, "Left"=w394:i32)
            n32 = Close Reference(reference=w393) -> ()  [unwired: 1 in, 1 out]
            n33 = call <vilib>:"VIAnUtil Get Terminal Data Type.vi"("error in (no error)"=w391, "Terminal"=w390) -> ("error out"=w387:errorcluster, "dup  Terminal"=w389:refnum<vi>, "Type Variant"=w388:variant)  [unwired: 6 in, 1 out]
            n34 = call <vilib>:"VIAnUtil Check Type If ErrClust.vi"("error in (no error)"=w387, "Data In"=w388) -> ("error out"=w392:errorcluster, "IsErrClust?"=w406:bool)  [unwired: 8 out]
            n35 = Not(x=w406) -> (.not. x?=w404:bool)
            n36 = for {
              tunnel: w395 -> [w423] mode=indexing
              tunnel: [w420] -> w401 mode=indexing
              tunnel: w392 -> [w414]
              w419 = refnum<vi> refnum  # GObject
              n37 = property class="Term"(reference=w423, error in=w414) -> (error out=w418:errorcluster, "Owner"=w422:refnum<vi>)  [unwired: 1 out]
              n38 = property class="Gen"(reference=w422, error in=w418) -> (reference out=w416:refnum<vi>, error out=w417:errorcluster, "Owner"=w421:refnum<vi>)
              n39 = Close Reference(reference=w416, error in (no error)=w417) -> (error out=w415:errorcluster)
              n40 = To More Specific Class(target class=w419, reference=w421, error in=w415) -> (specific class reference=w420:refnum<vi>)  [unwired: 1 out]
            }
            n41 = Bundle By Name(cluster=T1 {"Not Error Wire?"=FALSE, "Source Term Top"=0, "Source Term Left"=0, "Wire Ref"=refnum, "Source Term"=refnum, "Sink Terms"=[], "Tried this one yet?"=FALSE, "Sink Term Owner Owners"=[]} ("Wire Information"), "Not Error Wire?"=w404, "Source Term Top"=w405, "Source Term Left"=w394, "Wire Ref"=w403, "Source Term"=w389, "Sink Terms"=w395, "Tried this one yet?"=FALSE, "Sink Term Owner Owners"=w401) -> (w399:T1)
          }
          n42 = Sort 1D Array(array=w65) -> (sorted array=w68:T7)
          n43 = Close Reference(reference=w71, error in (no error)=w64) -> (error out=w63:errorcluster)
          n44 = case shown="False" w69 {
            tunnel: w63 -> [w81 w386]
            tunnel: w68 -> [w82 _]
            tunnel: [w80 w386] -> w60
            tunnel: w61 -> [w77 _]
            tunnel: w62 -> [w76 _]
            tunnel: [TRUE FALSE] -> w59
            tunnel: w58 -> [w74 _]
            tunnel: w57 -> [w73 _]
            tunnel: w56 -> [w72 _]
            frame False {
              w79 = refnum<vi> refnum  # Node
              n45 = while {
                shift-right: [w96] -> _
                shift-left: w82 -> [w93]
                shift-right: [w87] -> w78
                shift-left: w79 -> [w95]
                tunnel: w77 -> [w89]
                tunnel: w76 -> [w88]
                tunnel: w81 -> [w97]
                tunnel: [w86] -> w80
                tunnel: w74 -> [w85]
                tunnel: w73 -> [w84]
                tunnel: w72 -> [w83]
                i -> [w98]
                stop <- w90 stop-if-true
                # "Stop iterating once we've gone through all the wires, or if an error occurs"
                n46 = Delete From Array(array=w93, index=0) -> (deleted portion=w99:T1, array with subset deleted=w92:T7)  [unwired: 1 in]
                n47 = case shown="Default" w98 {
                  tunnel: w99 -> [w123 w218]
                  tunnel: w97 -> [w120 w237]
                  tunnel: w92 -> [w114 w226]
                  tunnel: [w110 w236] -> w87
                  tunnel: [w124 w225] -> w96
                  tunnel: w95 -> [_ w236]
                  tunnel: [w122 w229] -> w86
                  tunnel: w89 -> [w106 _]
                  tunnel: w88 -> [w107 _]
                  tunnel: w85 -> [w105 _]
                  tunnel: w84 -> [w101 _]
                  tunnel: w83 -> [w104 _]
                  frame 0 {
                    w112 = refnum<vi> refnum  # Node
                    # "On the first iteration, do the Insert.  If the wire is an error wire, make sure it has different terms after the insert.  If so, the inserted node had error terminals and it's all good.  If not, then this function did not have error terminals, so we'll need to reprocess the error wire later.  This is for cases like the Add primitive with Waveform inputs, that doesn't get error terminals until the waveforms are both wired up.  If the wire is not an error wire, then delete the created wires immediately after the insert.  This is because the insert may have put the object in the wrong place, i.e. with a Max & Min function, the insert method always puts the top wire on the bottom terminals, which is not what we want, so we delete the wire and re-wire it up the right way on later iterations."
                    n48 = Unbundle By Name(w123) -> ("Not Error Wire?"=w118:bool, "Wire Ref"=w121:refnum<vi>)
                    n49 = property class="Wire"(reference=w121, error in=w120) -> (reference out=w109:refnum<vi>, error out=w108:errorcluster, "Terms[]"=w119:refnum<vi>[])
                    n50 = case shown="\"\"" w106 {
                      selector: w106 -> [w129 _]
                      tunnel: w109 -> [w130 w140]
                      tunnel: w108 -> [w128 w139]
                      tunnel: [w127 w138] -> w102
                      tunnel: [w126 w137] -> w100
                      tunnel: w105 -> [_ w134]
                      tunnel: w104 -> [_ w135]
                      tunnel: w107 -> [_ w132]
                      tunnel: [w125 w133] -> w103
                      tunnel: w101 -> [_ w131]
                      frame Default {
                        n51 = invoke class="Wire" method="Insert Node"(reference=w130, error in=w128, "PaletteString"=w129) -> (reference out=w125:refnum<vi>, error out=w127:errorcluster, "Insert Node"=w126:refnum<vi>)  [unwired: 4 in, 4 out]
                      }
                      frame "" {
                        n52 = Not A Number/Path/Refnum?(number/path/refnum=w134) -> (NaN/Path/Refnum?=w136:bool)
                        n53 = case shown="False" w136 {
                          tunnel: w140 -> [w146 w161]
                          tunnel: w132 -> [w145 _]
                          tunnel: w139 -> [w144 w160]
                          tunnel: [w143 w159] -> w138
                          tunnel: [w142 w158] -> w137
                          tunnel: w135 -> [_ w154]
                          tunnel: w131 -> [_ w153]
                          tunnel: w134 -> [_ w152]
                          tunnel: [w141 w147] -> w133
                          frame True {
                            n54 = invoke class="Wire" method="Insert Node"(reference=w146, error in=w144, "Path"=w145) -> (reference out=w141:refnum<vi>, error out=w143:errorcluster, "Insert Node"=w142:refnum<vi>)  [unwired: 4 in, 4 out]
                          }
                          frame False {
                            w151 = refnum<vi> refnum  # Node
                            n55 = To More Specific Class(target class=w151, reference=w152) -> (specific class reference=w155:refnum<vi>)  [unwired: 1 in, 1 out]
                            n56 = property class="Node"(reference=w155) -> (reference out=w148:refnum<vi>, "Style"=w156:string)  [unwired: 1 in, 1 out]
                            n57 = Search 1D Array(1D array=w153, element=w156) -> (index of element=w157:i32)  [unwired: 1 in]
                            n58 = Index Array(array=w154, index=w157) -> (element=w149:cluster{"String":string, "Value":i32})
                            n59 = Greater Or Equal To 0?(x=w157) -> (x >= 0?=w150:bool)
                            n60 = case shown="True" w150 {
                              tunnel: w161 -> [w168 w177]
                              tunnel: w160 -> [w167 w176]
                              tunnel: [w166 w175] -> w159
                              tunnel: [w165 w174] -> w158
                              tunnel: w149 -> [w164 _]
                              tunnel: w148 -> [_ w173]
                              tunnel: [w162 w169] -> w147
                              frame True {
                                n61 = Unbundle By Name(w164) -> ("Value"=w163:i32)
                                n62 = invoke class="Wire" method="Insert Node"(reference=w168, error in=w167, "Style"=w163) -> (reference out=w162:refnum<vi>, error out=w166:errorcluster, "Insert Node"=w165:refnum<vi>)  [unwired: 4 in, 4 out]
                              }
                              frame False {
                                w171 = refnum<vi> refnum  # SubVI
                                n63 = To More Specific Class(target class=w171, reference=w173) -> (specific class reference=w172:refnum<vi>)  [unwired: 1 in, 1 out]
                                n64 = property class="SubVI"(reference=w172) -> ("VIPath"=w170:path)  [unwired: 1 in, 2 out]
                                n65 = invoke class="Wire" method="Insert Node"(reference=w177, error in=w176, "Path"=w170) -> (reference out=w169:refnum<vi>, error out=w175:errorcluster, "Insert Node"=w174:refnum<vi>)  [unwired: 4 in, 4 out]
                              }
                            }
                          }
                        }
                      }
                    }
                    n66 = property class="Wire"(reference=w103, error in=w102) -> (reference out=w117:refnum<vi>, error out=w113:errorcluster, "Broken?"=w116:bool)
                    n67 = Or(x=w118, y=w116) -> (x .or. y?=w115:bool)
                    n68 = To More Specific Class(target class=w112, reference=w100, error in=w113) -> (specific class reference=w110:refnum<vi>, error out=w111:errorcluster)
                    n69 = case shown="False" w115 {
                      tunnel: w114 -> [w185 w205]
                      tunnel: [w183 w204] -> w124
                      tunnel: w123 -> [w184 w203]
                      tunnel: [w178 w200] -> w122
                      tunnel: w111 -> [w180 w202]
                      tunnel: w117 -> [_ w201]
                      tunnel: w119 -> [_ w198]
                      tunnel: w110 -> [w181 _]
                      frame True {
                        n70 = property class="Node"(reference=w181, error in=w180) -> (error out=w182:errorcluster, "Terms[]"=w179:refnum<vi>[])  [unwired: 1 out]
                        n71 = Build Array (concatenate)(w184, w185) -> (w183:T7)
                        n72 = for {
                          shift-right: [w187] -> w178
                          shift-left: w182 -> [w193]
                          tunnel: w179 -> [w192] mode=indexing
                          n73 = property class="Term"(reference=w192, error in=w193) -> (reference out=w190:refnum<vi>, error out=w191:errorcluster, "Wire"=w186:refnum<vi>)
                          n74 = Close Reference(reference=w190, error in (no error)=w191) -> (error out=w188:errorcluster)
                          n75 = Not A Number/Path/Refnum?(number/path/refnum=w186) -> (NaN/Path/Refnum?=w189:bool)
                          n76 = case shown="False" w189 {
                            tunnel: w188 -> [w194 w196]
                            tunnel: [w194 w196] -> w187
                            tunnel: w186 -> [w195 _]
                            frame False {
                              n77 = invoke class="Wire" method="Delete"(reference=w195, error in=w194) -> ()  [unwired: 1 in, 3 out]
                            }
                            frame True {
                            }
                          }
                        }
                      }
                      frame False {
                        n78 = property class="Wire"(reference=w201, error in=w202) -> (error out=w200:errorcluster, "Terms[]"=w199:refnum<vi>[])  [unwired: 1 out]
                        n79 = Not Equal?(x=w198, y=w199) -> (x != y?=w197:bool)
                        n80 = case shown="False" w197 {
                          tunnel: w205 -> [w210 w211]
                          tunnel: [w209 w211] -> w204
                          tunnel: w203 -> [w208 _]
                          frame False {
                            n81 = Bundle By Name(cluster=w208, "Tried this one yet?"=TRUE) -> (w207:T1)
                            n82 = Build Array (concatenate)(w210, w207) -> (w209:T7)
                          }
                          frame True {
                          }
                        }
                      }
                    }
                  }
                  frame Default {
                    # "If we haven't tried this wire before, and we weren't able to wire it, then add it to the end of the list so we can try it one more time before giving up.  This is for Nodes whose terminals change as things are wired to them.  But if we have tried this one already, don't add it to the list again, just give up on it."
                    # "Try to wire up this wire's source term to one of the inputs of the Node, starting with the top ones.  If the created wire is broken, this isn't a compatible data type, so delete it.  If the created wire is not broken, then this is a valid connection.  Clean up the wire, and stop the loop."
                    # "We need to read the Terms[] on the Node each iteration, as they may have changed as a result of things being wired (like the Add pac-man).  This code gets position information for each terminal on the node and sorts the info, so we can attempt to do the smart insert on unwired terminals starting from the top down."
                    n83 = property class="Node"(reference=w236, error in=w237) -> (error out=w234:errorcluster, "Terms[]"=w235:refnum<vi>[])  [unwired: 1 out]
                    n84 = Initialize Array(T1 {"Not Error Wire?"=FALSE, "Source Term Top"=0, "Source Term Left"=0, "Wire Ref"=refnum, "Source Term"=refnum, "Sink Terms"=[], "Tried this one yet?"=FALSE, "Sink Term Owner Owners"=[]} ("Wire Information"), 0) -> (w212:T7)
                    n85 = for {
                      tunnel: w235 -> [w343] mode=indexing
                      shift-right: [w336] -> w219
                      shift-left: w234 -> [w344]
                      shift-right: [w339] -> w232
                      shift-left: w212 -> [w342]
                      shift-right: [w338] -> w230
                      shift-left: w212 -> [w340]
                      n86 = property class="Term"(reference=w343, error in=w344) -> (reference out=w334:refnum<vi>, error out=w337:errorcluster, "Wire"=w335:refnum<vi>)
                      n87 = Not A Number/Path/Refnum?(number/path/refnum=w335) -> (NaN/Path/Refnum?=w341:bool)
                      n88 = case shown="True" w341 {
                        tunnel: w342 -> [w350 w357]
                        tunnel: w340 -> [w349 w356]
                        tunnel: [w350 w354] -> w339
                        tunnel: [w349 w355] -> w338
                        tunnel: w337 -> [w347 w360]
                        tunnel: [w346 w351] -> w336
                        tunnel: w335 -> [w348 _]
                        tunnel: w334 -> [w345 w359]
                        frame False {
                          n89 = Close Reference(reference=w345, error in (no error)=w347) -> (error out=w346:errorcluster)
                          n90 = Close Reference(reference=w348) -> ()  [unwired: 1 in, 1 out]
                        }
                        frame True {
                          n91 = property class="Term"(reference=w359, error in=w360) -> (reference out=w353:refnum<vi>, error out=w352:errorcluster, "IsSource"=w358:bool)
                          n92 = case shown="True" w358 {
                            tunnel: w357 -> [w370 w382]
                            tunnel: w356 -> [w371 w384]
                            tunnel: [w371 w383] -> w355
                            tunnel: [w369 w382] -> w354
                            tunnel: w353 -> [w366 w381]
                            tunnel: w352 -> [w362 w373]
                            tunnel: [w361 w372] -> w351
                            frame False {
                              n93 = property class="Term"(reference=w366, error in=w362) -> (reference out=w363:refnum<vi>, error out=w361:errorcluster, "Left"=w365:i32, "Top"=w364:i32)
                              n94 = Bundle By Name(cluster=T1 {"Not Error Wire?"=FALSE, "Source Term Top"=0, "Source Term Left"=0, "Wire Ref"=refnum, "Source Term"=refnum, "Sink Terms"=[], "Tried this one yet?"=FALSE, "Sink Term Owner Owners"=[]} ("Wire Information"), "Source Term Left"=w365, "Source Term Top"=w364, "Source Term"=w363) -> (w367:T1)
                              n95 = Build Array (concatenate)(w370, w367) -> (w369:T7)
                            }
                            frame True {
                              n96 = property class="Term"(reference=w381, error in=w373) -> (reference out=w378:refnum<vi>, error out=w372:errorcluster, "Left"=w375:i32, "Top"=w377:i32)
                              n97 = Subtract(x=99999, y=w375) -> (x-y=w374:i32)
                              n98 = Bundle By Name(cluster=T1 {"Not Error Wire?"=FALSE, "Source Term Top"=0, "Source Term Left"=0, "Wire Ref"=refnum, "Source Term"=refnum, "Sink Terms"=[], "Tried this one yet?"=FALSE, "Sink Term Owner Owners"=[]} ("Wire Information"), "Source Term Left"=w374, "Source Term Top"=w377, "Source Term"=w378) -> (w379:T1)
                              n99 = Build Array (concatenate)(w384, w379) -> (w383:T7)
                            }
                          }
                        }
                      }
                    }
                    n100 = Unbundle By Name(w218) -> ("Sink Terms"=w217:refnum<vi>[], "Sink Term Owner Owners"=w216:refnum<vi>[], "Source Term"=w214:refnum<vi>, "Wire Ref"=w213:refnum<vi>)
                    n101 = Sort 1D Array(array=w232) -> (sorted array=w224:T7)
                    n102 = Sort 1D Array(array=w230) -> (sorted array=w223:T7)
                    n103 = Empty Array?(array=w223) -> (empty?=w215:bool)
                    n104 = Not A Number/Path/Refnum?(number/path/refnum=w213) -> (NaN/Path/Refnum?=w222:bool)
                    n105 = case shown="False" w222 {
                      tunnel: w219 -> [w238 w240]
                      tunnel: [w238 w240] -> w233
                      tunnel: w213 -> [w239 _]
                      frame False {
                        n106 = invoke class="Wire" method="Delete"(reference=w239, error in=w238) -> ()  [unwired: 1 in, 3 out]
                      }
                      frame True {
                      }
                    }
                    n107 = for {
                      tunnel: w214 -> [w324]
                      tunnel: w224 -> [w323] mode=indexing
                      shift-right: [w316] -> w231
                      shift-left: w233 -> [w325]
                      tunnel: [w315] -> w227
                      stop <- w315 continue-if-true
                      n108 = Unbundle By Name(w323) -> ("Source Term"=w314:refnum<vi>)
                      n109 = invoke class="Term" method="Connect Wire"(reference=w324, error in=w325, "Wire Source"=w314) -> (reference out=w321:refnum<vi>, error out=w322:errorcluster)  [unwired: 4 in, 5 out]
                      n110 = property class="Term"(reference=w321, error in=w322) -> (error out=w320:errorcluster, "Wire"=w319:refnum<vi>)  [unwired: 1 out]
                      n111 = property class="Wire"(reference=w319, error in=w320) -> (reference out=w317:refnum<vi>, error out=w318:errorcluster, "Broken?"=w315:bool)
                      n112 = case shown="False" w315 {
                        tunnel: w318 -> [w330 w332]
                        tunnel: w317 -> [w329 w333]
                        tunnel: [w326 w331] -> w316
                        frame False {
                          n113 = invoke class="Wire" method="CleanUpWire"(reference=w329, error in=w330) -> (reference out=w327:refnum<vi>, error out=w328:errorcluster)  [unwired: 1 in, 1 out]
                          n114 = Close Reference(reference=w327, error in (no error)=w328) -> (error out=w326:errorcluster)
                        }
                        frame True {
                          n115 = invoke class="Wire" method="Delete"(reference=w333, error in=w332) -> (error out=w331:errorcluster)  [unwired: 1 in, 2 out]
                        }
                      }
                    }
                    n116 = case shown="False" w215 {
                      tunnel: w231 -> [w256 w302]
                      tunnel: w217 -> [w255 _]
                      tunnel: [w249 w302] -> w229
                      tunnel: [w248 w301] -> w228
                      tunnel: w227 -> [w246 w301]
                      tunnel: w216 -> [w244 _]
                      tunnel: w223 -> [w241 _]
                      frame False {
                        # "Same as before, but with Node output terminals.  Since the selected wire may have had more than one sink, try to wire the first one to the node's output.  If it works, the following loop does the rest of them."
                        n117 = Delete From Array(array=w255, index=0) -> (deleted portion=w253:refnum<vi>, array with subset deleted=w250:refnum<vi>[])  [unwired: 1 in]
                        n118 = Delete From Array(array=w244, index=0) -> (deleted portion=w243:refnum<vi>, array with subset deleted=w242:refnum<vi>[])  [unwired: 1 in]
                        n119 = for {
                          tunnel: w253 -> [w278]
                          tunnel: w241 -> [w283] mode=indexing
                          shift-right: [w285] -> w252
                          shift-left: w256 -> [w292]
                          tunnel: [w280] -> w247
                          tunnel: [w281] -> w251
                          tunnel: w243 -> [w284]
                          tunnel: [w277] -> _
                          stop <- w280 continue-if-true
                          n120 = Unbundle By Name(w283) -> ("Source Term"=w281:refnum<vi>)
                          n121 = property class="Term"(reference=w278) -> (error out=w279:errorcluster, "ClassName"=w277:string)  [unwired: 1 in, 1 out]
                          n122 = Select(t=w284, s=w279, f=w278) -> (s? t:f=w282:refnum<vi>)
                          n123 = invoke class="Term" method="Connect Wire"(reference=w281, error in=w292, "Wire Source"=w282) -> (reference out=w290:refnum<vi>, error out=w291:errorcluster)  [unwired: 4 in, 5 out]
                          n124 = property class="Term"(reference=w290, error in=w291) -> (error out=w289:errorcluster, "Wire"=w288:refnum<vi>)  [unwired: 1 out]
                          n125 = property class="Wire"(reference=w288, error in=w289) -> (reference out=w286:refnum<vi>, error out=w287:errorcluster, "Broken?"=w280:bool)
                          n126 = case shown="False" w280 {
                            tunnel: w287 -> [w297 w299]
                            tunnel: w286 -> [w296 w300]
                            tunnel: [w293 w298] -> w285
                            frame False {
                              n127 = invoke class="Wire" method="CleanUpWire"(reference=w296, error in=w297) -> (reference out=w294:refnum<vi>, error out=w295:errorcluster)  [unwired: 1 in, 1 out]
                              n128 = Close Reference(reference=w294, error in (no error)=w295) -> (error out=w293:errorcluster)
                            }
                            frame True {
                              n129 = invoke class="Wire" method="Delete"(reference=w300, error in=w299) -> (error out=w298:errorcluster)  [unwired: 1 in, 2 out]
                            }
                          }
                        }
                        n130 = case shown="False" w247 {
                          tunnel: w252 -> [w261 w276]
                          tunnel: [w258 w276] -> w249
                          tunnel: w251 -> [w260 _]
                          tunnel: w250 -> [w259 _]
                          tunnel: w242 -> [w257 _]
                          frame False {
                            n131 = for {
                              tunnel: w260 -> [w274]
                              tunnel: w259 -> [w263] mode=indexing
                              shift-right: [w267] -> w258
                              shift-left: w261 -> [w275]
                              tunnel: w257 -> [w266] mode=indexing
                              tunnel: [w262] -> _
                              # "Connecting the first sink terminalto the node worked, so go ahead and connect the rest."
                              n132 = property class="Term"(reference=w263) -> (error out=w264:errorcluster, "ClassName"=w262:string)  [unwired: 1 in, 1 out]
                              n133 = Select(t=w266, s=w264, f=w263) -> (s? t:f=w265:refnum<vi>)
                              n134 = invoke class="Term" method="Connect Wire"(reference=w274, error in=w275, "Wire Source"=w265) -> (reference out=w273:refnum<vi>, error out=w272:errorcluster)  [unwired: 4 in, 5 out]
                              n135 = property class="Term"(reference=w273, error in=w272) -> (error out=w271:errorcluster, "Wire"=w270:refnum<vi>)  [unwired: 1 out]
                              n136 = invoke class="Wire" method="CleanUpWire"(reference=w270, error in=w271) -> (reference out=w268:refnum<vi>, error out=w269:errorcluster)  [unwired: 1 in, 1 out]
                              n137 = Close Reference(reference=w268, error in (no error)=w269) -> (error out=w267:errorcluster)
                            }
                          }
                          frame True {
                            # "None of the node outputs would connect to this wire.  No need to try to process the rest of the sinks."
                          }
                        }
                        n138 = And(x=w247, y=w246) -> (x .and. y?=w248:bool)
                      }
                      frame True {
                        # "There are no more unwired outputs on the node.  Don't bother trying to find one to wire to."
                      }
                    }
                    n139 = case shown="True" w228 {
                      tunnel: w226 -> [w303 w307]
                      tunnel: w218 -> [_ w304]
                      tunnel: [w303 w305] -> w225
                      frame False {
                      }
                      frame True {
                        n140 = Unbundle By Name(w304) -> ("Tried this one yet?"=w306:bool)
                        n141 = case shown="False" w306 {
                          tunnel: w307 -> [w312 w313]
                          tunnel: [w311 w313] -> w305
                          tunnel: w304 -> [w310 _]
                          frame False {
                            n142 = Bundle By Name(cluster=w310, "Tried this one yet?"=TRUE) -> (w309:T1)
                            n143 = Build Array (concatenate)(w312, w309) -> (w311:T7)
                          }
                          frame True {
                          }
                        }
                      }
                    }
                  }
                }
                n144 = Empty Array?(array=w96) -> (empty?=w91:bool)
                n145 = Or(x=w91, y=w86) -> (x .or. y?=w90:bool)
              }
              n146 = Close Reference(reference=w78) -> ()  [unwired: 1 in, 1 out]
            }
            frame True {
              # "The wires weren't all on the same diagram.  This is a no-op."
            }
          }
        }
        frame True {
          # "If multiple items were inserted, see if they all have the same insert position (within 5 pixels of each other).  If so, then tile them so they don't overlap."
          # "Do a standard insert on each selected wire.  If any of the Inserts return with no error, then we want to complete the Undo transaction.  If they all errored out, then we'll fail the Undo transaction."
          n147 = for {
            tunnel: w441 -> [w522]
            tunnel: w440 -> [w521]
            tunnel: w439 -> [w496] mode=indexing
            shift-right: [w519] -> w437
            shift-left: FALSE -> [w520]
            tunnel: w432 -> [w517]
            tunnel: [w518] -> w434 mode=indexing
            tunnel: w431 -> [w501]
            tunnel: w430 -> [w499]
            tunnel: w429 -> [w500]
            tunnel: w428 -> [w498] mode=indexing
            w511 = i16 2 ("y")
            # "See if there is a selected wire segment. If so, calculate the midpoint of the segment and specify that as the InsertPoint. If there is not a selected segment, then do a normal insert (i.e. with no InsertPoint specified)."
            n148 = Unbundle(w498) -> ("Joints[]"=w497:T4)
            n149 = for {
              tunnel: w497 -> [w655] mode=indexing
              tunnel: w497 -> [w654]
              tunnel: [w655] -> w506
              tunnel: [w653] -> w507
              tunnel: [w643] -> w503
              stop <- w643 stop-if-true
              # "If selected is T, and either SelectedRight or SelectedDown is T, then the joint is actually selected."
              # "Flag 3 - Selected?\nFlag 4 - SelectedRight?\nFlag 5 - SelectedDown?"
              n150 = Unbundle By Name(w655) -> ("Up Joint Index"=w650:i16, "Left Joint Index"=w649:i16, "Down Joint Index"=w652:i16, "Right Joint Index"=w651:i16, "Flags"=w661:i32)
              n151 = Number To Boolean Array(number=w661) -> (Boolean array=w660:bool[])
              n152 = Index Array(array=w660, index #1=3 ("index")) -> (element #1=w656:bool, element #2=w657:bool, element #3=w648:bool)  [unwired: 2 in]
              n153 = Select(t=w650, s=w648, f=w649) -> (s? t:f=w645:i16)
              n154 = Or(x=w657, y=w648) -> (x .or. y?=w658:bool)
              n155 = Select(t=w652, s=w648, f=w651) -> (s? t:f=w644:i16)
              n156 = Less Than 0?(x=w644) -> (x < 0?=w646:bool)
              n157 = And(x=w656, y=w658) -> (x .and. y?=w643:bool)
              n158 = Select(t=w645, s=w646, f=w644) -> (s? t:f=w647:i16)
              n159 = Index Array(array=w654, index=w647) -> (element=w653:T8)
            }
            n160 = Unbundle By Name(w506) -> ("Position.h"=w513:i16, "Position.v"=w515:i16)
            n161 = Unbundle By Name(w507) -> ("Position.h"=w514:i16, "Position.v"=w516:i16)
            n162 = Add(x=w513, y=w514) -> (x+y=w508:i16)
            n163 = Add(x=w515, y=w516) -> (x+y=w510:i16)
            n164 = Quotient & Remainder(x=w508, y=w511) -> (floor(x/y)=w509:i16)  [unwired: 1 out]
            n165 = Quotient & Remainder(x=w510, y=w511) -> (floor(x/y)=w512:i16)  [unwired: 1 out]
            n166 = Bundle(cluster=T3 {"Horizontal"=0, "Vertical"=0} ("Insertion Point"), "Horizontal"=w509, "Vertical"=w512) -> (w502:T3)
            n167 = case shown="False" w503 {
              tunnel: w522 -> [w532 w595]
              tunnel: w521 -> [w531 w594]
              tunnel: [w530 w593] -> w518
              tunnel: w496 -> [w529 w592]
              tunnel: w517 -> [w528 w591]
              tunnel: [w527 w590] -> w504
              tunnel: w502 -> [w526 w589]
              tunnel: w501 -> [w525 w588]
              tunnel: w500 -> [w524 w587]
              tunnel: w499 -> [w523 w586]
              frame True {
                n168 = case shown="\"\"" w532 {
                  selector: w532 -> [w537 _]
                  tunnel: w529 -> [w538 w548]
                  tunnel: w531 -> [_ w540]
                  tunnel: w528 -> [w536 w547]
                  tunnel: [w535 w546] -> w527
                  tunnel: [w534 w545] -> w530
                  tunnel: w526 -> [w533 w544]
                  tunnel: w525 -> [_ w541]
                  tunnel: w524 -> [_ w543]
                  tunnel: w523 -> [_ w542]
                  frame Default {
                    n169 = invoke class="Wire" method="Insert Node"(reference=w538, error in=w536, "PaletteString"=w537, "InsertPoint"=w533) -> (error out=w535:errorcluster, "Insert Node"=w534:refnum<vi>)  [unwired: 3 in, 5 out]
                  }
                  frame "" {
                    n170 = Not A Number/Path/Refnum?(number/path/refnum=w541) -> ()  [unwired: 1 out]
                    n171 = Empty String/Path?(string/path=w540) -> (empty?=w539:bool)
                    n172 = case shown="False" w539 {
                      tunnel: w548 -> [w563 w585]
                      tunnel: w540 -> [_ w584]
                      tunnel: w547 -> [w562 w583]
                      tunnel: [w561 w582] -> w546
                      tunnel: [w560 w581] -> w545
                      tunnel: w544 -> [w559 w580]
                      tunnel: w543 -> [w555 _]
                      tunnel: w542 -> [w554 _]
                      tunnel: w541 -> [w553 _]
                      frame True {
                        w552 = refnum<vi> refnum  # Node
                        n173 = To More Specific Class(target class=w552, reference=w553) -> (specific class reference=w556:refnum<vi>)  [unwired: 1 in, 1 out]
                        n174 = property class="Node"(reference=w556) -> (reference out=w549:refnum<vi>, "Style"=w557:string)  [unwired: 1 in, 1 out]
                        n175 = Search 1D Array(1D array=w554, element=w557) -> (index of element=w558:i32)  [unwired: 1 in]
                        n176 = Index Array(array=w555, index=w558) -> (element=w550:cluster{"String":string, "Value":i32})
                        n177 = Greater Or Equal To 0?(x=w558) -> (x >= 0?=w551:bool)
                        n178 = case shown="False" w551 {
                          tunnel: w563 -> [w570 w579]
                          tunnel: w562 -> [w569 w578]
                          tunnel: [w568 w577] -> w561
                          tunnel: [w567 w576] -> w560
                          tunnel: w559 -> [w566 w575]
                          tunnel: w550 -> [w565 _]
                          tunnel: w549 -> [_ w574]
                          frame True {
                            n179 = Unbundle By Name(w565) -> ("Value"=w564:i32)
                            n180 = invoke class="Wire" method="Insert Node"(reference=w570, error in=w569, "Style"=w564, "InsertPoint"=w566) -> (error out=w568:errorcluster, "Insert Node"=w567:refnum<vi>)  [unwired: 3 in, 5 out]
                          }
                          frame False {
                            w572 = refnum<vi> refnum  # SubVI
                            n181 = To More Specific Class(target class=w572, reference=w574) -> (specific class reference=w573:refnum<vi>)  [unwired: 1 in, 1 out]
                            n182 = property class="SubVI"(reference=w573) -> ("VIPath"=w571:path)  [unwired: 1 in, 2 out]
                            n183 = invoke class="Wire" method="Insert Node"(reference=w579, error in=w578, "Path"=w571, "InsertPoint"=w575) -> (error out=w577:errorcluster, "Insert Node"=w576:refnum<vi>)  [unwired: 3 in, 5 out]
                          }
                        }
                      }
                      frame False {
                        n184 = invoke class="Wire" method="Insert Node"(reference=w585, error in=w583, "Path"=w584, "InsertPoint"=w580) -> (error out=w582:errorcluster, "Insert Node"=w581:refnum<vi>)  [unwired: 3 in, 5 out]
                      }
                    }
                  }
                }
              }
              frame False {
                n185 = case shown="\"\"" w595 {
                  selector: w595 -> [w599 _]
                  tunnel: w592 -> [w600 w609]
                  tunnel: w594 -> [_ w602]
                  tunnel: w591 -> [w598 w608]
                  tunnel: [w597 w607] -> w590
                  tunnel: [w596 w606] -> w593
                  tunnel: w589 -> [_ _]
                  tunnel: w588 -> [_ w603]
                  tunnel: w587 -> [_ w605]
                  tunnel: w586 -> [_ w604]
                  frame Default {
                    n186 = invoke class="Wire" method="Insert Node"(reference=w600, error in=w598, "PaletteString"=w599) -> (error out=w597:errorcluster, "Insert Node"=w596:refnum<vi>)  [unwired: 4 in, 5 out]
                  }
                  frame "" {
                    n187 = Not A Number/Path/Refnum?(number/path/refnum=w603) -> ()  [unwired: 1 out]
                    n188 = Empty String/Path?(string/path=w602) -> (empty?=w601:bool)
                    n189 = case shown="True" w601 {
                      tunnel: w609 -> [w623 w642]
                      tunnel: w602 -> [_ w641]
                      tunnel: w608 -> [w622 w640]
                      tunnel: [w621 w639] -> w607
                      tunnel: [w620 w638] -> w606
                      tunnel: w605 -> [w616 _]
                      tunnel: w604 -> [w615 _]
                      tunnel: w603 -> [w614 _]
                      frame True {
                        w613 = refnum<vi> refnum  # Node
                        n190 = To More Specific Class(target class=w613, reference=w614) -> (specific class reference=w617:refnum<vi>)  [unwired: 1 in, 1 out]
                        n191 = property class="Node"(reference=w617) -> (reference out=w610:refnum<vi>, "Style"=w618:string)  [unwired: 1 in, 1 out]
                        n192 = Search 1D Array(1D array=w615, element=w618) -> (index of element=w619:i32)  [unwired: 1 in]
                        n193 = Index Array(array=w616, index=w619) -> (element=w611:cluster{"String":string, "Value":i32})
                        n194 = Greater Or Equal To 0?(x=w619) -> (x >= 0?=w612:bool)
                        n195 = case shown="True" w612 {
                          tunnel: w623 -> [w629 w637]
                          tunnel: w622 -> [w628 w636]
                          tunnel: [w627 w635] -> w621
                          tunnel: [w626 w634] -> w620
                          tunnel: w611 -> [w625 _]
                          tunnel: w610 -> [_ w633]
                          frame True {
                            n196 = Unbundle By Name(w625) -> ("Value"=w624:i32)
                            n197 = invoke class="Wire" method="Insert Node"(reference=w629, error in=w628, "Style"=w624) -> (error out=w627:errorcluster, "Insert Node"=w626:refnum<vi>)  [unwired: 4 in, 5 out]
                          }
                          frame False {
                            w631 = refnum<vi> refnum  # SubVI
                            n198 = To More Specific Class(target class=w631, reference=w633) -> (specific class reference=w632:refnum<vi>)  [unwired: 1 in, 1 out]
                            n199 = property class="SubVI"(reference=w632) -> ("VIPath"=w630:path)  [unwired: 1 in, 2 out]
                            n200 = invoke class="Wire" method="Insert Node"(reference=w637, error in=w636, "Path"=w630) -> (error out=w635:errorcluster, "Insert Node"=w634:refnum<vi>)  [unwired: 4 in, 5 out]
                          }
                        }
                      }
                      frame False {
                        n201 = invoke class="Wire" method="Insert Node"(reference=w642, error in=w640, "Path"=w641) -> (error out=w639:errorcluster, "Insert Node"=w638:refnum<vi>)  [unwired: 4 in, 5 out]
                      }
                    }
                  }
                }
              }
            }
            n202 = Compound Arithmetic op=OR(invert w504, w520) -> (w519:bool)
          }
          n203 = for {
            shift-right: [w444] -> w436
            shift-left: w432 -> [w447]
            tunnel: w434 -> [w443] mode=indexing
            shift-right: [w446] -> _
            shift-left: T2[] [] -> [w445]
            n204 = Not A Number/Path/Refnum?(number/path/refnum=w443) -> (NaN/Path/Refnum?=w442:bool)
            n205 = case shown="True" w442 {
              tunnel: w447 -> [w456 w495]
              tunnel: w443 -> [w455 _]
              tunnel: [w453 w494] -> w446
              tunnel: w445 -> [w450 w494]
              tunnel: [w451 w495] -> w444
              frame False {
                # "See if current item's position is within 5 pixels of any other item's position."
                n206 = property class="GObj"(reference=w455, error in=w456) -> (reference out=w452:refnum<vi>, error out=w454:errorcluster, "Position"=w449:T2)
                n207 = for {
                  tunnel: w450 -> [w465] mode=indexing
                  tunnel: w449 -> [w461]
                  tunnel: [w457] -> w448
                  stop <- w457 stop-if-true
                  w464 = 5 ("y")
                  n208 = Add(x=w465, y=w464) -> (x+y=w463:T2)
                  n209 = Subtract(x=w465, y=w464) -> (x-y=w462:T2)
                  n210 = In Range and Coerce(upper limit=w463, x=w461, lower limit=w462) -> (In Range?=w460:cluster{"Left":bool, "Top":bool})  [unwired: 1 out]
                  n211 = Unbundle(w460) -> ("Left"=w459:bool, "Top"=w458:bool)
                  n212 = And(x=w459, y=w458) -> (x .and. y?=w457:bool)
                }
                n213 = case shown="True" w448 {
                  tunnel: w450 -> [w469 w493]
                  tunnel: [w468 w492] -> w453
                  tunnel: w449 -> [w467 w491]
                  tunnel: w454 -> [w471 w490]
                  tunnel: w452 -> [w472 _]
                  tunnel: [w470 w490] -> w451
                  frame True {
                    # "This object position exists (within 5 pixels of another object). Add 5 pixels to h/v until a position is found that does not overlap (with 5 pixels), and use that."
                    n214 = while {
                      tunnel: w469 -> [w475]
                      tunnel: w467 -> [w476]
                      tunnel: [w474] -> w466
                      i -> [w480]
                      stop <- w473 continue-if-true
                      # "See if current item's position is within 5 pixels of any other item's position."
                      n215 = Increment(x=w480) -> (x+1=w479:i32)
                      n216 = Multiply(x=5 ("y"), y=w479) -> (x*y=w477:i32)
                      n217 = Add(x=w476, y=w477) -> (x+y=w474:T2)
                      n218 = for {
                        tunnel: w475 -> [w489] mode=indexing
                        tunnel: w474 -> [w485]
                        tunnel: [w481] -> w473
                        stop <- w481 stop-if-true
                        w488 = 5 ("y")
                        n219 = Add(x=w489, y=w488) -> (x+y=w487:T2)
                        n220 = Subtract(x=w489, y=w488) -> (x-y=w486:T2)
                        n221 = In Range and Coerce(upper limit=w487, x=w485, lower limit=w486) -> (In Range?=w484:cluster{"Left":bool, "Top":bool})  [unwired: 1 out]
                        n222 = Unbundle(w484) -> ("Left"=w483:bool, "Top"=w482:bool)
                        n223 = And(x=w483, y=w482) -> (x .and. y?=w481:bool)
                      }
                    }
                    n224 = property class="GObj"(reference=w472, error in=w471, "Position"=w466) -> (error out=w470:errorcluster)  [unwired: 1 out]
                    n225 = Build Array (concatenate)(w469, w466) -> (w468:T2[])
                  }
                  frame False {
                    # "This object's position doesn't exist in the array. Store it to compare with later objects."
                    n226 = Build Array (concatenate)(w493, w491) -> (w492:T2[])
                  }
                }
              }
              frame True {
                # "Invalid refnum...don't bother doing anything"
              }
            }
          }
          n227 = Close Reference(reference=w434, error in (no error)=w436) -> (error out=w435:errorcluster)
        }
      }
      n228 = case shown="True" w21 {
        tunnel: w19 -> [w678 w681]
        tunnel: [w679 w682] -> w33
        tunnel: w22 -> [_ _]
        tunnel: w13 -> [w677 _]
        frame True {
          n229 = invoke class="VI" method="Transaction.End Undo"(reference=w678) -> (error out=w679:errorcluster)  [unwired: 2 in, 2 out]
          n230 = for {
            tunnel: w677 -> [w680] mode=indexing
            n231 = invoke class="GObj" method="Delete"(reference=w680) -> ()  [unwired: 2 in, 3 out]
          }
        }
        frame False {
          n232 = invoke class="VI" method="Transaction.Fail"(reference=w681) -> (error out=w682:errorcluster)  [unwired: 2 in, 2 out]
        }
      }
    }
    frame Error {
    }
  }
  "error out" <- w6
  "Variant out" <- w1
